vi "Puff Dose Low.vi"(0 "Save Puff Analysis file":bool, 1 "Row Number":i32, 2 "Valve Index":i32, 3 "File Extension":string=".xls", 5 "Puff Stats only?":bool, 9 "Save individual puff files":bool, 11 "Analysis info Cluster in":T2={"Colour"=0, "Inst type"=enum."Propeller anemometer", "Inst name"="", "Symbol"="", "Code name"="", "Extra Info"="", "Inst Array"=enum."PWA", "U"=0.0, "u^2"=0.0, "u^3"=0.0, "u^4"=0.0, "Skew_u"=0.0, "Kurt_u"=0.0, "Sd Error in Mean"=0.0, "% u'/U"=0.0, "X"=0.0, "Y"=0.0, "Z"=0.0, "Timescale integral Estimate"=0.0, "Sd Error in Variance"=0.0, "Calib File"=path "", "Calib Constants"=[], "Output Position"=FALSE, "Stats"=enum."None", "Av Sampling Rate"=0.0, "Av No of Samples"=0.0, "Total Meas Time (s)"=0.0, "OrigChName"="", "Max value"=0.0, "Min value"=0.0, "Req Sample Rate Hz"=0.0, "Sync Delay Time (s)"=0.0, "Ch No"=0, "Device"="", "Use Latest Calib"=FALSE, "Port"="", "Metadata Ch Names"=[], "Metadata Ch Values"=[], "Label"="", "chState"=enum."Solo", "Point Drift"=0.0, "inputConfig"=""} {"Kurt_u" format="%_3g"; "u^4" format="%_3g"; "u^3" format="%_3g"; "Sd Error in Variance" format="%_3g"; "u^2" format="%_3g"; "Sd Error in Mean" format="%_3g"; "U" format="%_3g"; "Sync Delay Time (s)" format="%.4f"; "Total Meas Time (s)" format="%_5g"; "Skew_u" format="%_3g"; "% u'/U" format="%_3g"}, 12 "Saved trace length":i32=200, 13 "FFID Index":i32, 14 "Save Av puff files":bool) -> (4 "File to Update":T1[](array[typedef]), 15 "Analysis info Cluster out":T2={"Colour"=0, "Inst type"=enum."Propeller anemometer", "Inst name"="", "Symbol"="", "Code name"="", "Extra Info"="", "Inst Array"=enum."PWA", "U"=0.0, "u^2"=0.0, "u^3"=0.0, "u^4"=0.0, "Skew_u"=0.0, "Kurt_u"=0.0, "Sd Error in Mean"=0.0, "% u'/U"=0.0, "X"=0.0, "Y"=0.0, "Z"=0.0, "Timescale integral Estimate"=0.0, "Sd Error in Variance"=0.0, "Calib File"=path "", "Calib Constants"=[], "Output Position"=FALSE, "Stats"=enum."None", "Av Sampling Rate"=0.0, "Av No of Samples"=0.0, "Total Meas Time (s)"=0.0, "OrigChName"="", "Max value"=0.0, "Min value"=0.0, "Req Sample Rate Hz"=0.0, "Sync Delay Time (s)"=0.0, "Ch No"=0, "Device"="", "Use Latest Calib"=FALSE, "Port"="", "Metadata Ch Names"=[], "Metadata Ch Values"=[], "Label"="", "chState"=enum."Solo", "Point Drift"=0.0, "inputConfig"=""} {"Kurt_u" format="%_3g"; "u^4" format="%_3g"; "u^3" format="%_3g"; "Sd Error in Variance" format="%_3g"; "u^2" format="%_3g"; "Sd Error in Mean" format="%_3g"; "U" format="%_3g"; "Sync Delay Time (s)" format="%.4f"; "Total Meas Time (s)" format="%_5g"; "Skew_u" format="%_3g"; "% u'/U" format="%_3g"})   [LabVIEW 2022 SP3]
uses:
  Controls/Analysis_info_cluster.ctl
  Controls/Inst_type.ctl
  Controls/Instrument_Array.ctl
  Controls/channelState.ctl
  File/File Update Cluster.ctl
  <vilib>/Analysis/baseanly.llb/Mean (DBL).vi
  Globals/Meas_global.vi
  Globals/Plug_in_data_global.vi
  Globals/Dynamic_call_global.ph.vi
  <vilib>/Analysis/NI_AALBase.lvlib
  <vilib>/Analysis/NI_AALPro.lvlib
panel:
  in  "Time constants cut off":dbl=3.0
  out "Numeric":dbl
  out "End Index":i32
  out "Start Index":i32
  out "Av Dose below Threshold":dbl format="%0.2f"
  out "Max Flight Time (s)":dbl
  out "Table Control":string[][](table)
  out "Minimum Dose":dbl
  out "Initial Minimum Dose":dbl
  out "Active Length":i32
  out "T1 index":i32
  out "Initial Time of Flight":dbl
  out "Output:Data File:Location":string
  out "Dose per Puff":cluster{dbl[], "Best Polynomial Fit":dbl[]}[](graph)
  out "Polynomial Coefficients":dbl[](array[numeric])
  out "Bkgnd Per Puff":cluster{dbl[], "Best Polynomial Fit":dbl[]}[](graph)
  out "Background time used (s)":dbl
  out "Delta T":dbl
  out "Bkgnd value (ppm)":dbl format="%0.2f"
  out "Puff Number":i32=51
  out "XY Graph":cluster{"Time (s)":dbl[], "Eng Values":dbl[]}[](graph)
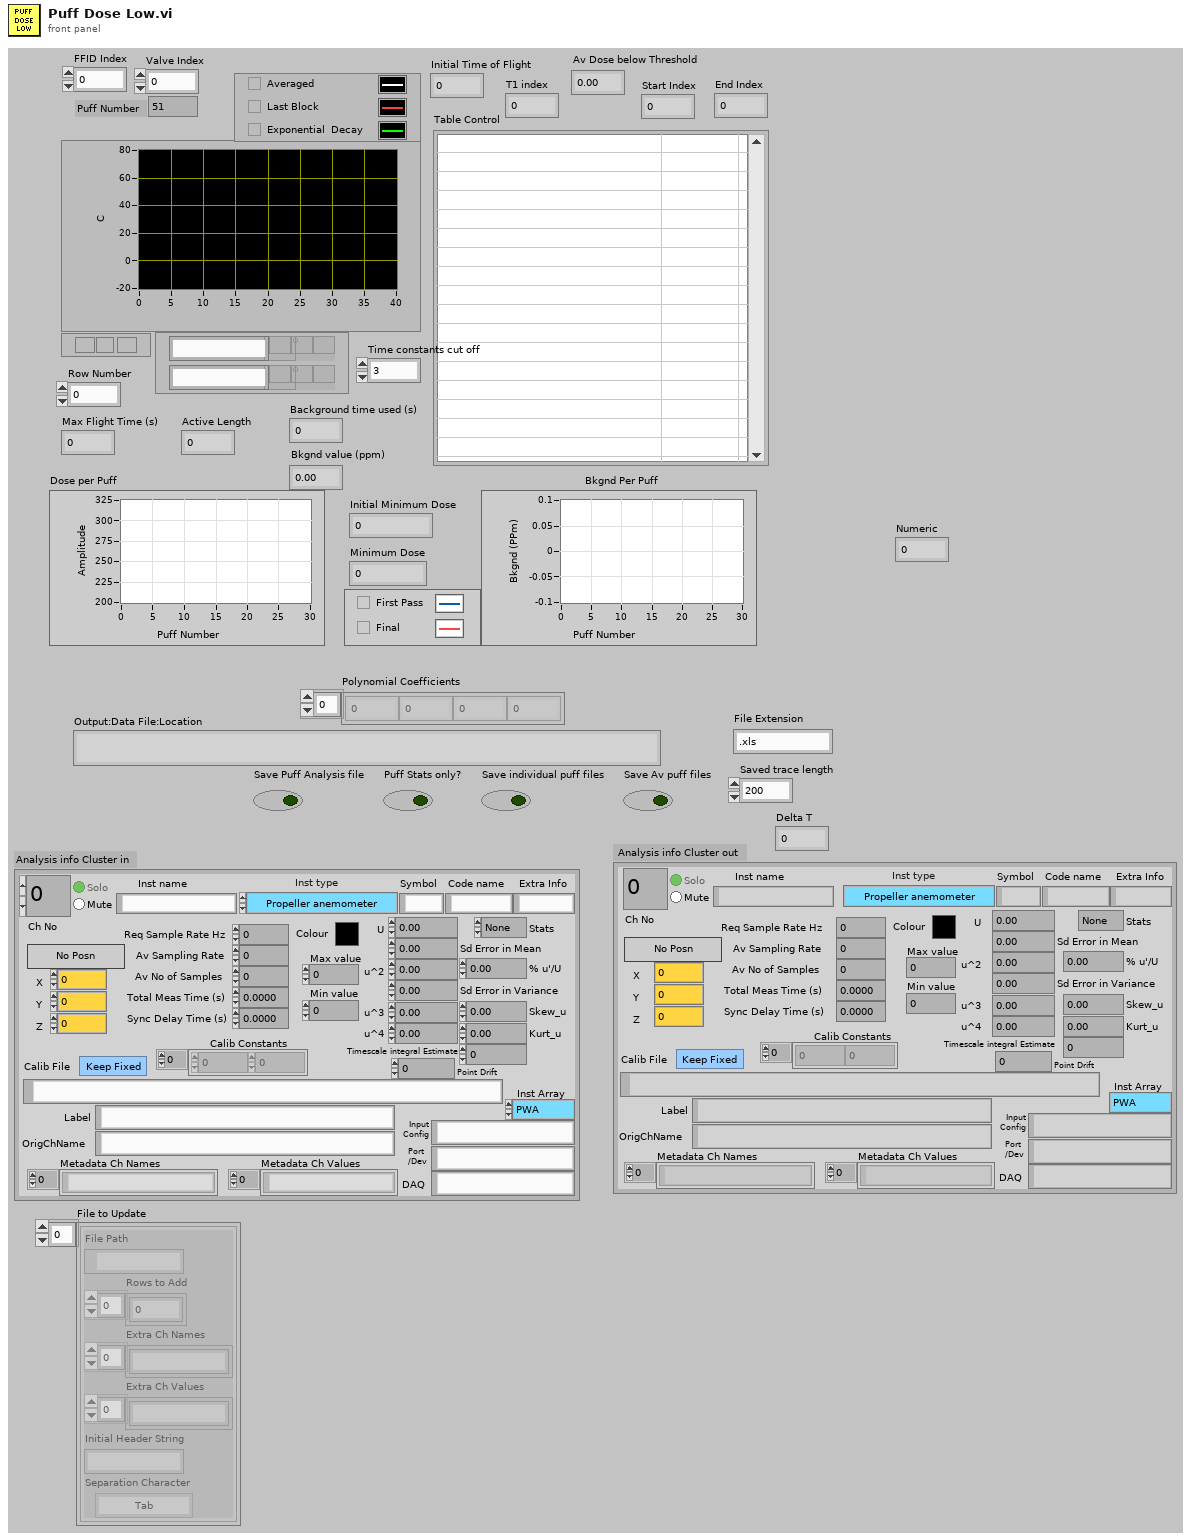
[diagram p1: front panel]
types:
  T1 = typedef "File Update Cluster.ctl" = cluster{"File Path":path, "Rows to Add":i32[], "Extra Ch Names":string[], "Extra Ch Values":string[], "Initial Header String":string, "Separation Character":enum16{"Tab", "Comma"}}
  T2 = typedef "Analysis_info_cluster.ctl" = cluster{"Colour":u32, "Inst type":T3, "Inst name":string, "Symbol":string, "Code name":string, "Extra Info":string, "Inst Array":T4, "U":dbl, "u^2":dbl, "u^3":dbl, "u^4":dbl, "Skew_u":dbl, "Kurt_u":dbl, "Sd Error in Mean":dbl, "% u'/U":dbl, "X":dbl, "Y":dbl, "Z":dbl, "Timescale integral Estimate":dbl, "Sd Error in Variance":dbl, "Calib File":path, "Calib Constants":dbl[], "Output Position":bool, "Stats":enum16{"None", "Basic", "Full"}, "Av Sampling Rate":dbl, "Av No of Samples":dbl, "Total Meas Time (s)":dbl, "OrigChName":string, "Max value":dbl, "Min value":dbl, "Req Sample Rate Hz":dbl, "Sync Delay Time (s)":dbl, "Ch No":i16, "Device":string, "Use Latest Calib":bool, "Port":string, "Metadata Ch Names":string[], "Metadata Ch Values":string[], "Label":string, "chState":T5, "Point Drift":dbl, "inputConfig":string}
  T3 = typedef "Inst_type.ctl" = enum16{"Raw voltage", "Raw with zero offsetting", "Propeller anemometer", "Pressure Transducer", "Pitot-static tube", "Hot wire", "Cross wire 1", "Cross wire 2", "Generic Linear", "Generic Polynomial", "Generic BackPoly", "Fast FID", "Thermocouple", "Cold wire", "Pulsed Wire", "LDA Vel", "LDA Tran time", "LDA Arr time", "Microphone"}
  T4 = typedef "Instrument_Array.ctl" = enum16{"PWA", "LDA", "Analogue"}
  T5 = typedef "channelState.ctl" = enum32{"No Selection", "Solo", "Mute"}
  T6 = enum16{"Save no data", "Save data in new files", "Save data in existing files"}
  T7 = typedef "Time_Trace_Cluster.ctl" = cluster{"Weighting":dbl[], "Voltage":dbl[], "Eng Values":dbl[]}
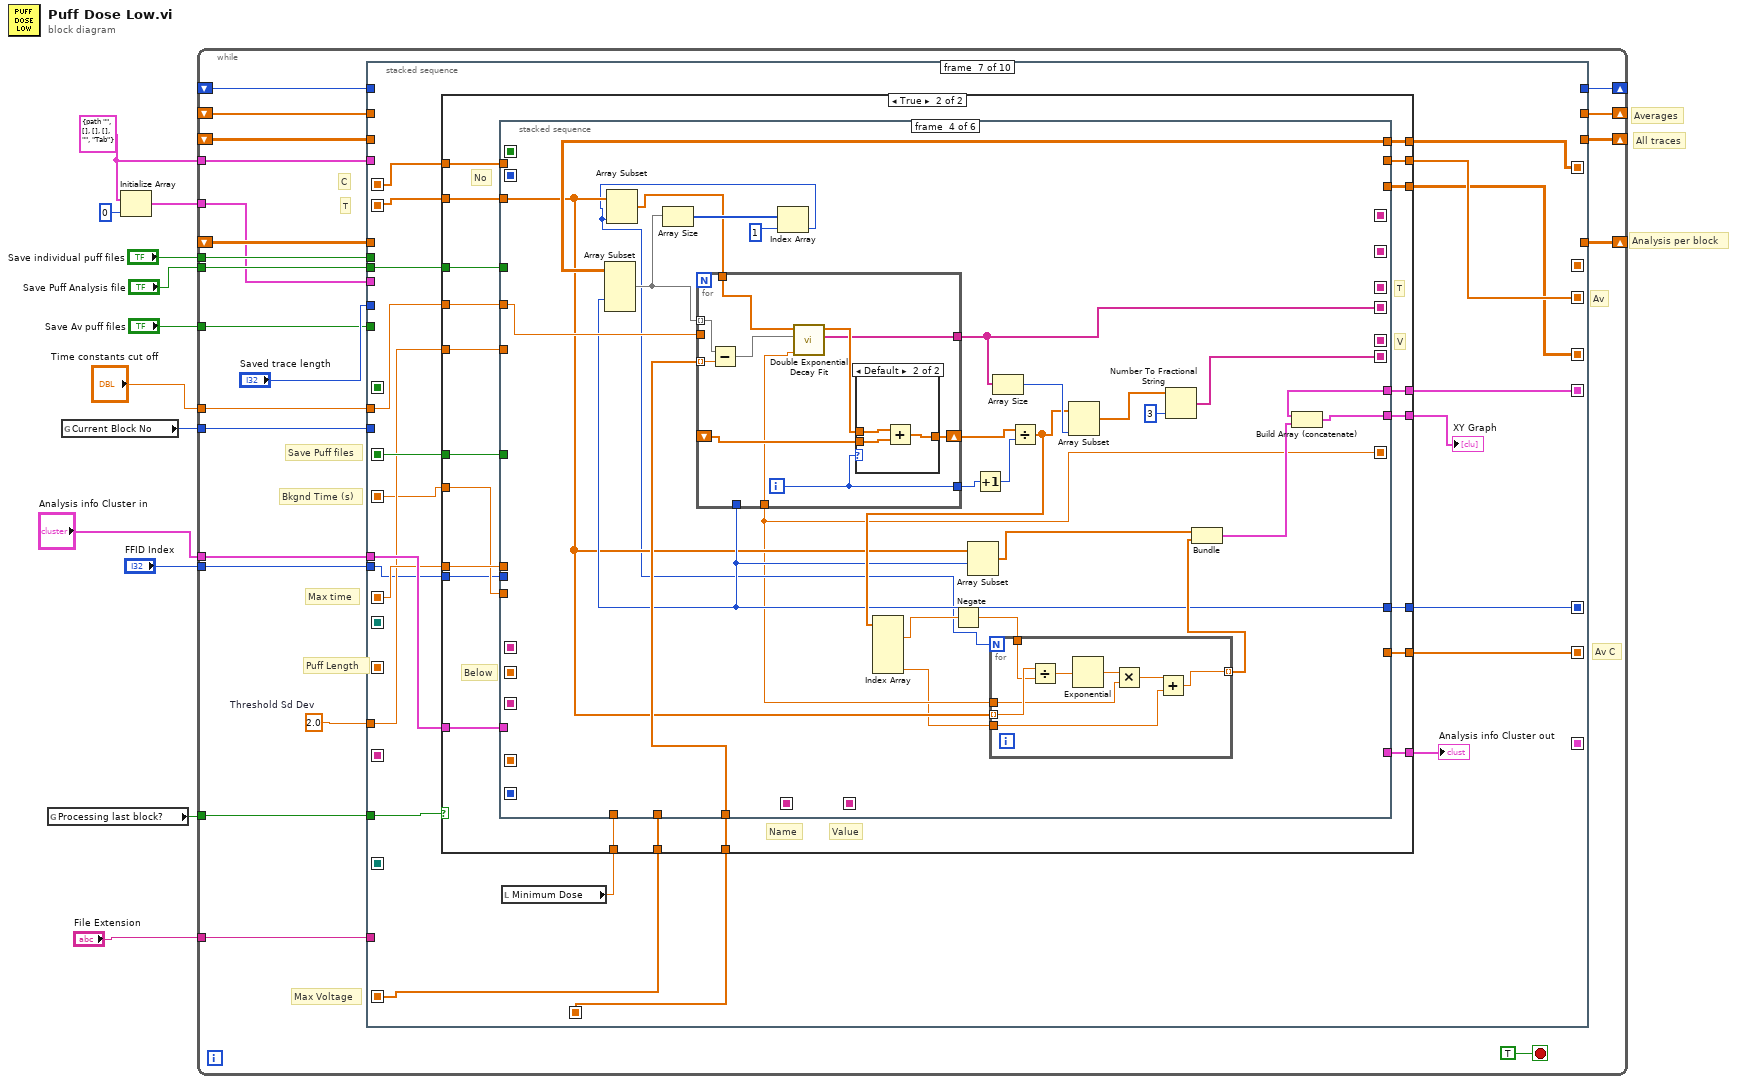
[diagram p0: block diagram]
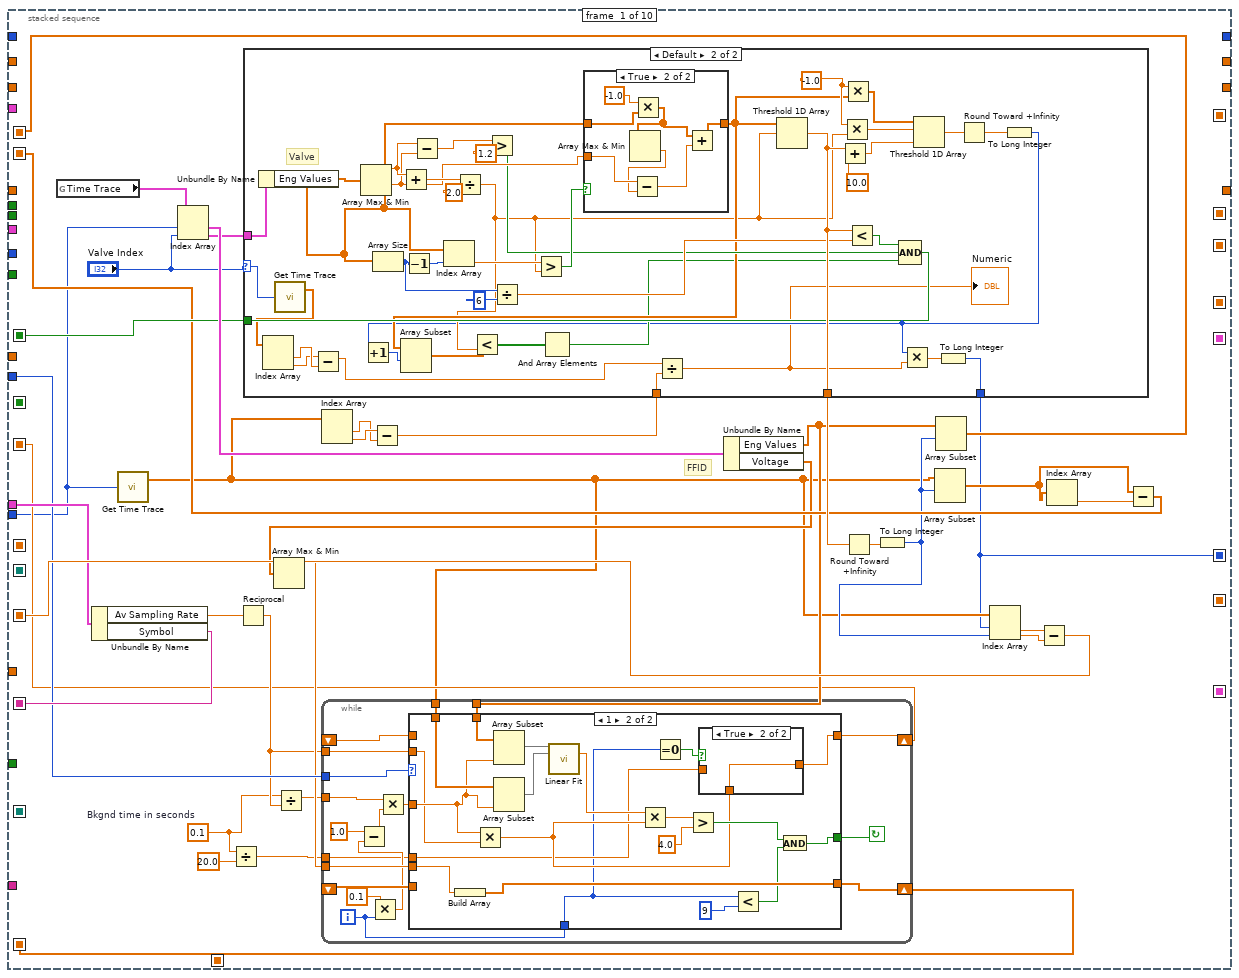
[diagram p2: hidden frame]
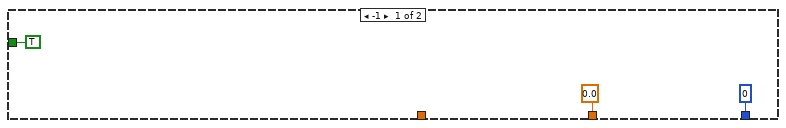
[diagram p3: hidden frame]
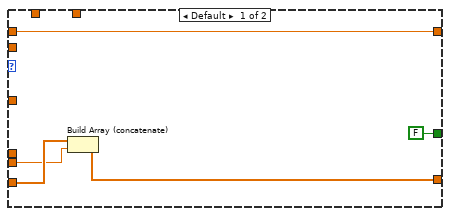
[diagram p5: hidden frame]
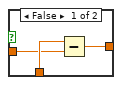
[diagram p6: hidden frame]
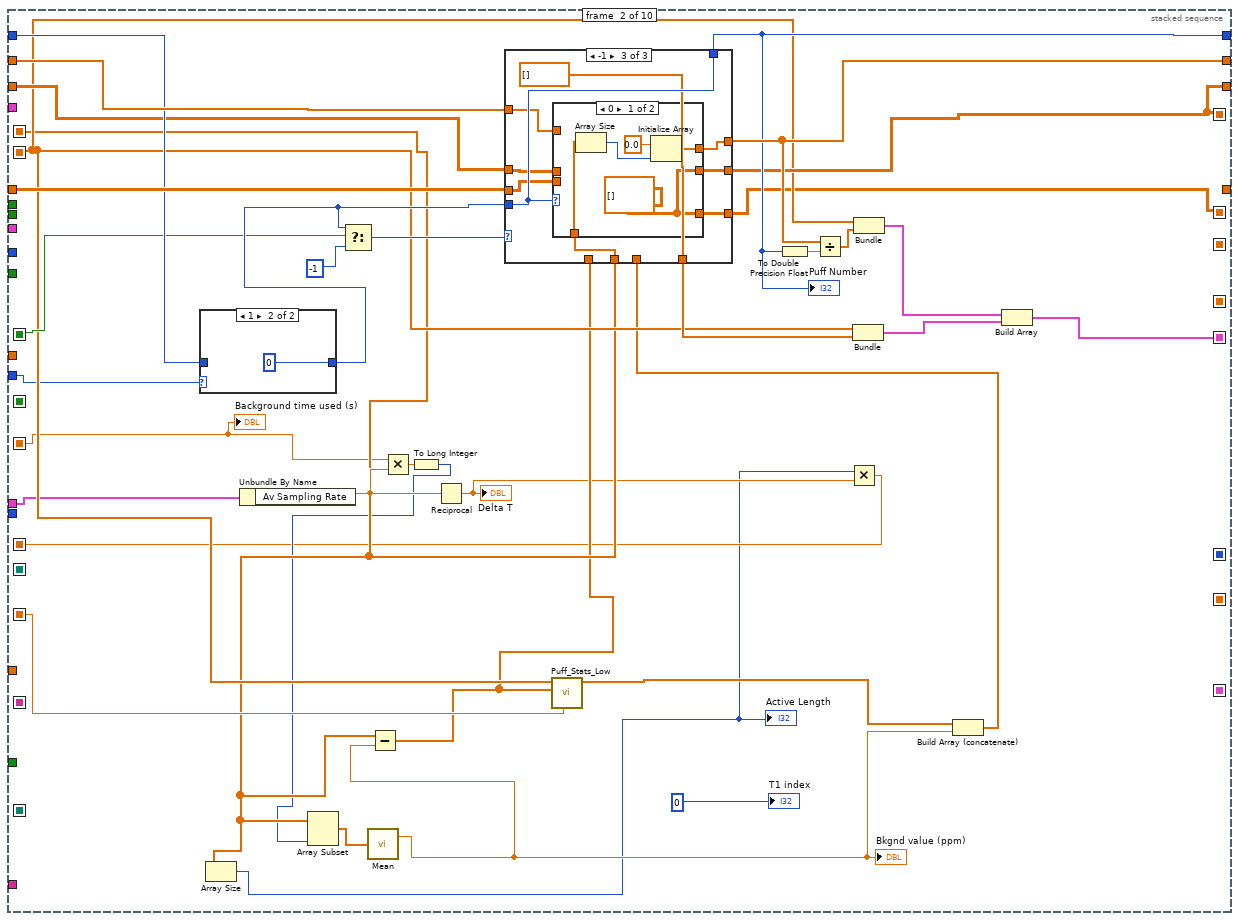
[diagram p7: hidden frame]
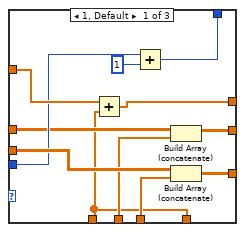
[diagram p9: hidden frame]
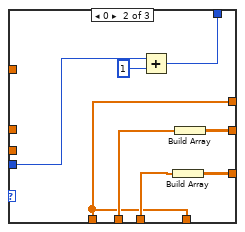
[diagram p10: hidden frame]
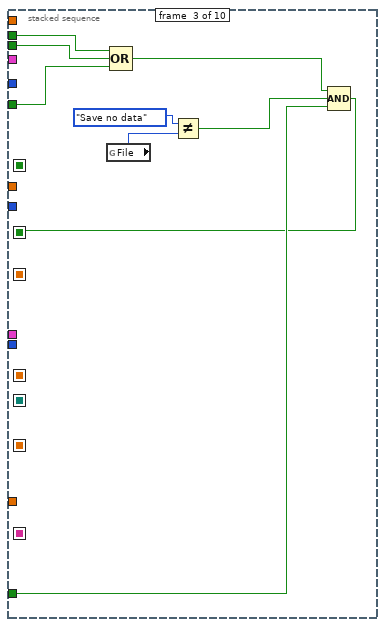
[diagram p12: hidden frame]
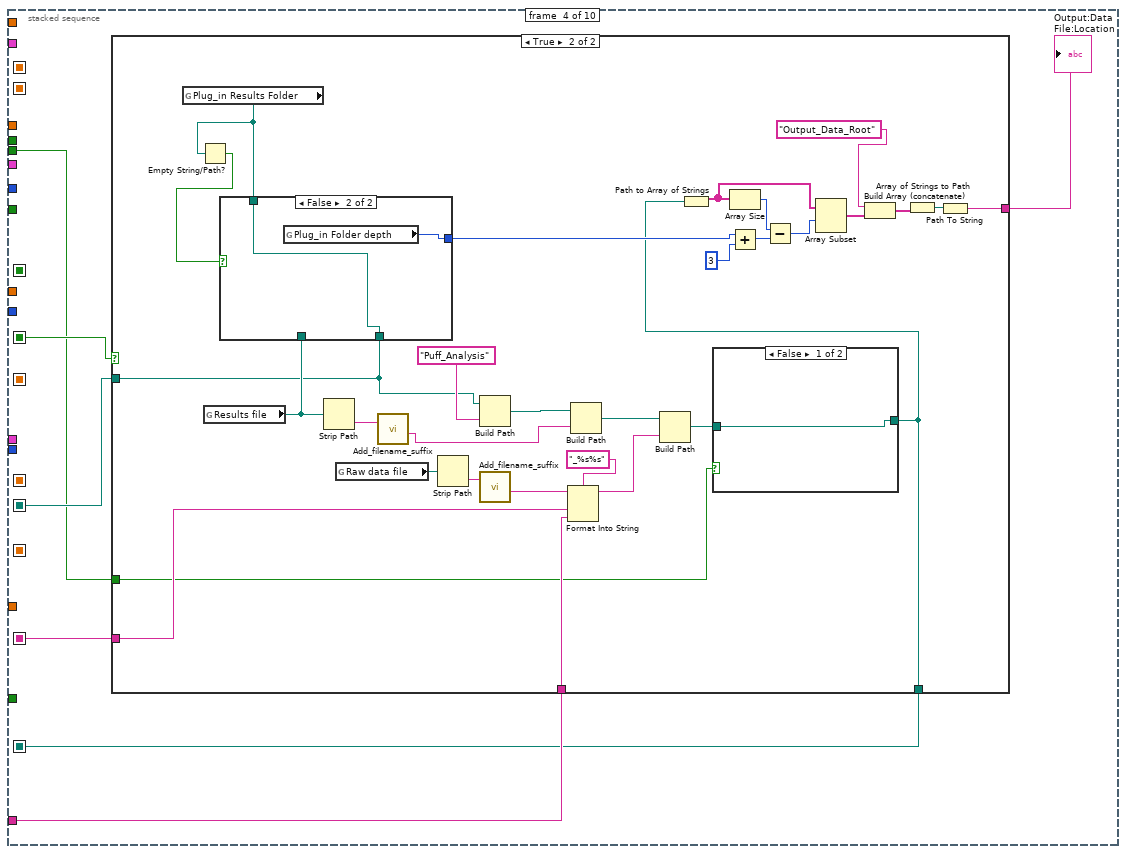
[diagram p13: hidden frame]
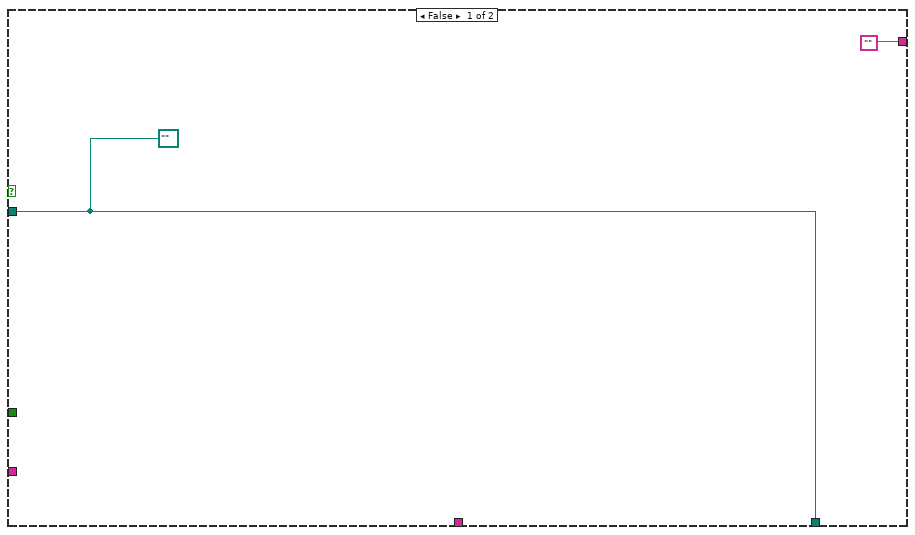
[diagram p14: hidden frame]
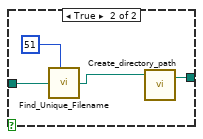
[diagram p15: hidden frame]
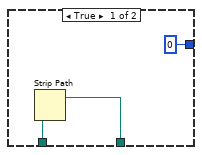
[diagram p16: hidden frame]
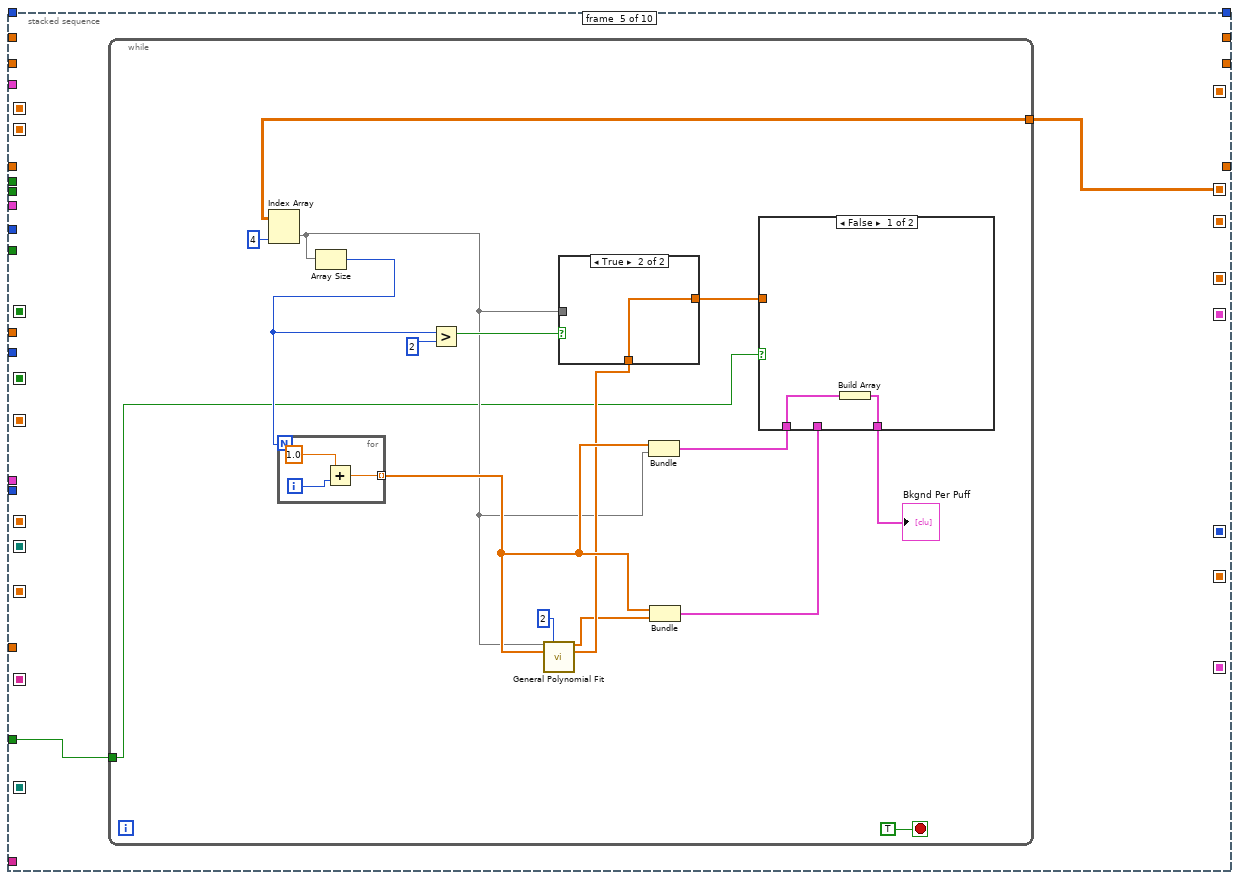
[diagram p17: hidden frame]
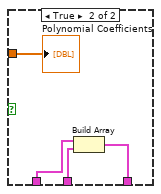
[diagram p18: hidden frame]
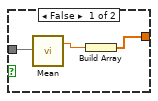
[diagram p19: hidden frame]
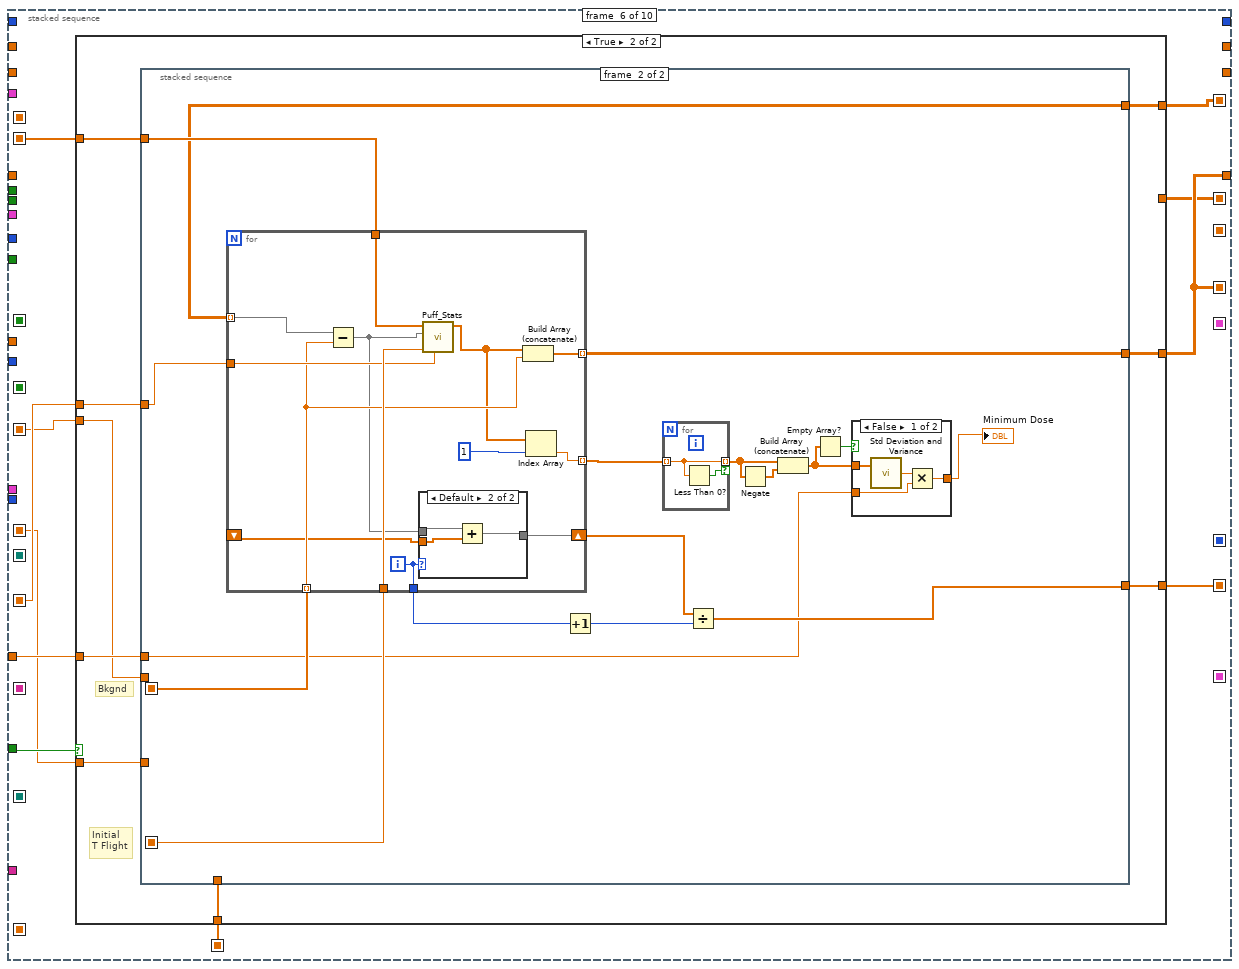
[diagram p20: hidden frame]
diagram:
  w2 = T1 {"File Path"=path "", "Rows to Add"=[], "Extra Ch Names"=[], "Extra Ch Values"=[], "Initial Header String"="", "Separation Character"=enum."Tab"} ("File to Update")
  # "Averages"
  # "All traces"
  # "Analysis per block"
  n1 = global read "Meas_global.vi" "Processing last block?"() -> (w11:bool)
  n2 = global read "Meas_global.vi" "Current Block No"() -> (w7:i32)
  n3 = Initialize Array(w2, 0 ("dimension size")) -> (w3:T1[])
  n4 = while {
    shift-right: [w32] -> _
    shift-left: _ -> [w34]
    shift-right: [w30] -> _
    shift-left: _ -> [w31]
    shift-right: [w28] -> _
    shift-left: _ -> [w29]
    shift-right: [w27] -> _
    shift-left: _ -> [w26]
    tunnel: "Save Puff Analysis file" -> [w25]
    tunnel: w11 -> [w24]
    tunnel: "FFID Index" -> [w23]
    tunnel: "Analysis info Cluster in" -> [w22]
    tunnel: "File Extension" -> [w21]
    tunnel: w7 -> [w19]
    tunnel: "Save Av puff files" -> [w17]
    tunnel: "Save individual puff files" -> [w16]
    tunnel: w3 -> [w15]
    tunnel: w2 -> [w14]
    tunnel: "Time constants cut off" -> [w13]
    stop <- TRUE stop-if-true
    w18 = 2.0  # Threshold Sd Dev
    # "Bkgnd Time (s)"
    # "Max time"
    # "Av C"
    # "Max Voltage"
    # "Av"
    # "Save Puff files"
    # "Puff Length"
    # "T"
    # "C"
    n5 = stacked-sequence {
      seq-local: [_ w178 _ _ _ _ _ _ _ _] -> [_ _ _ _ w303 w338 _ w698 _ _]
      seq-local: [w60 _ _ _ _ _ _ _ _ _] -> [_ w177 _ _ _ _ w451 _ _ _]
      seq-local: [w61 _ _ _ _ _ _ _ _ _] -> [_ w186 _ _ _ w341 w464 _ w728 _]
      seq-local: [w58 _ _ _ _ _ _ _ _ _] -> [_ w185 _ _ _ w340 _ _ _ _]
      seq-local: [w64 _ _ _ _ _ _ _ _ _] -> [_ w192 _ _ _ _ _ _ _ _]
      seq-local: [_ w188 _ _ _ _ _ _ _ _] -> [_ _ _ _ _ w342 w447 _ w729 _]
      seq-local: [_ _ w248 _ _ _ _ _ _ _] -> [_ _ _ w254 _ _ w460 _ w727 _]
      seq-local: [w59 _ _ _ _ _ _ _ _ _] -> [_ _ _ w258 _ _ _ _ w726 _]
      seq-local: [_ _ _ _ _ _ w463 _ _ _] -> [_ _ _ _ _ _ _ _ w724 _]
      seq-local: [_ _ _ w257 _ _ _ _ _ _] -> [_ _ _ _ _ _ _ _ w721 _]
      seq-local: [_ _ _ w255 _ _ _ _ _ _] -> [_ _ _ _ _ _ _ _ w722 _]
      seq-local: [_ _ _ _ _ _ _ _ w720 _] -> [_ _ _ _ _ _ _ _ _ w1015]
      seq-local: [w51 _ _ _ _ _ _ _ _ _] -> [_ _ _ _ _ _ w459 _ _ _]
      seq-local: [_ _ _ _ _ w339 _ _ _ _] -> [_ _ _ _ _ _ w458 w708 w718 _]
      seq-local: [_ _ _ _ _ w337 _ _ _ _] -> [_ _ _ _ _ _ w445 _ _ _]
      seq-local: [_ _ _ _ _ w336 _ _ _ _] -> [_ _ _ _ _ _ w456 _ w717 _]
      seq-local: [_ w172 _ _ _ _ _ _ _ _] -> [_ _ _ _ _ w334 w455 _ _ _]
      seq-local: [w45 _ _ _ _ _ _ _ _ _] -> [_ w170 _ _ _ w333 w453 _ _ _]
      seq-local: [w35 _ _ _ _ _ _ _ _ _] -> [_ _ _ _ _ _ w450 _ _ _]
      seq-local: [_ w169 _ _ _ _ _ _ _ _] -> [_ _ _ _ _ _ w449 _ _ _]
      tunnel: w34 -> [_ w198 _ _ _ _ _ _ _ _]
      tunnel: [_ w203 _ _ _ _ _ _ _ _] -> w32
      tunnel: w31 -> [_ w199 _ _ _ _ _ _ _ _]
      tunnel: [_ _ _ _ _ w339 _ _ _ _] -> w30
      tunnel: w29 -> [_ w197 _ _ _ _ _ _ _ _]
      tunnel: [_ w196 _ _ _ _ _ _ _ _] -> w28
      tunnel: [_ w188 _ _ _ _ _ _ _ _] -> w27
      tunnel: w26 -> [_ w190 _ _ _ _ _ _ _ _]
      tunnel: w25 -> [_ _ w246 w253 _ _ w466 _ w714 _]
      tunnel: w24 -> [_ _ w249 _ w302 w343 w465 _ _ _]
      tunnel: w17 -> [_ _ w245 _ _ _ _ _ w725 _]
      tunnel: w23 -> [w41 _ _ _ _ _ w452 _ _ _]
      tunnel: w22 -> [w54 w180 _ _ _ _ w462 _ w713 _]
      tunnel: w21 -> [_ _ _ w259 _ _ _ _ w723 _]
      tunnel: "Saved trace length" -> [_ _ _ _ _ _ _ _ w719 _]
      tunnel: w19 -> [w53 w179 _ _ _ _ _ _ _ _]
      tunnel: w18 -> [_ _ _ _ _ w335 w454 _ _ _]
      tunnel: w16 -> [_ _ w247 _ _ _ _ _ w716 _]
      tunnel: w15 -> [_ _ _ _ _ _ _ _ w715 _]
      tunnel: w14 -> [_ _ _ _ _ _ _ _ w712 _]
      tunnel: w13 -> [_ _ _ _ _ _ w446 _ _ _]
      frame #0 {
        w44 = 0.1  # Bkgnd time in seconds
        # "FFID"
        n6 = global read "Meas_global.vi" "Time Trace"() -> (w69:T7[])
        n7 = Unbundle By Name(w54) -> ("Av Sampling Rate"=w48:dbl, "Symbol"=w59:string)
        n8 = call "Get Time Trace.vi"("Channel Index"=w41) -> ("Time (s)"=w39:dbl[])  [unwired: 1 out]
        n9 = Index Array(array=w69, index #1=w41, index #2="Valve Index") -> (element #1=w68:T7, element #2=w67:T7)
        n10 = Divide(x=w44, y=20.0) -> (x/y=w42:dbl)
        n11 = Reciprocal(x=w48) -> (1/x=w46:dbl)
        n12 = Divide(x=w44, y=w46) -> (x/y=w47:dbl)
        n13 = Index Array(array=w39) -> (element #1=w37:dbl, element #2=w38:dbl)  [unwired: 2 in]
        n14 = Subtract(x=w38, y=w37) -> (x-y=w36:dbl)
        n15 = case shown="Default" "Valve Index" {
          selector: "Valve Index" -> [_ w82]
          tunnel: w67 -> [_ w113]
          tunnel: [0.0 w98] -> w65
          tunnel: [TRUE w92] -> w64
          tunnel: [0 w74] -> w35
          tunnel: w36 -> [_ w77]
          frame -1 {
          }
          frame Default {
            w108 = -1.0
            # "Valve"
            n16 = Unbundle By Name(w113) -> ("Eng Values"=w91:dbl[])
            n17 = call "Get Time Trace.vi"("Channel Index"=w82) -> ("Time (s)"=w79:dbl[])  [unwired: 1 out]
            n18 = Index Array(array=w79) -> (element #1=w81:dbl, element #2=w80:dbl)  [unwired: 2 in]
            n19 = Subtract(x=w80, y=w81) -> (x-y=w78:dbl)
            n20 = Array Max & Min(array=w91) -> (max value=w102:dbl, min value=w101:dbl)  [unwired: 2 out]
            n21 = Array Size(array=w91) -> (size(s)=w97:i32)
            n22 = Add(x=w102, y=w101) -> (x+y=w112:dbl)
            n23 = Decrement(x=w97) -> (x-1=w106:i32)
            n24 = Subtract(x=w102, y=w101) -> (x-y=w100:dbl)
            n25 = Index Array(array=w91, index=w106) -> (element=w105:dbl)
            n26 = Divide(x=w112, y=2.0) -> (x/y=w87:dbl)
            n27 = Greater?(x=w100, y=1.2) -> (0:w93:bool)
            n28 = Divide(x=w97, y=6) -> (x/y=w95:dbl)
            n29 = Greater?(x=w105, y=w87) -> (0:w104:bool)
            n30 = case shown="True" w104 {
              tunnel: w91 -> [w114 w120]
              tunnel: [w114 w115] -> w89
              tunnel: w101 -> [_ w119]
              frame False {
              }
              frame True {
                n31 = Multiply(x=-1.0, y=w120) -> (x*y=w116:dbl[])
                n32 = Array Max & Min(array=w116) -> (min value=w118:dbl)  [unwired: 3 out]
                n33 = Subtract(x=w119, y=w118) -> (x-y=w117:dbl)
                n34 = Add(x=w116, y=w117) -> (x+y=w115:dbl[])
              }
            }
            n35 = Divide(x=w78, y=w77) -> (x/y=w73:dbl)
            "Numeric" <- w73
            n36 = Threshold 1D Array(2:w87, 3:w89) -> (0:w98:dbl)  [unwired: 1 in]
            n37 = Add(x=w98, y=10.0) -> (x+y=w110:dbl)
            n38 = Multiply(x=w108, y=w87) -> (x*y=w107:dbl)
            n39 = Multiply(x=w108, y=w89) -> (x*y=w103:dbl[])
            n40 = Less?(x=w98, y=w95) -> (x < y?=w94:bool)
            n41 = Threshold 1D Array(1:w110, 2:w107, 3:w103) -> (0:w84:dbl)
            n42 = Round Toward +Infinity(x=w84) -> (ceil(x): smallest int >= x=w83:dbl)
            n43 = To Long Integer(number=w83) -> (32bit integer=w76:i32)
            n44 = Increment(x=w76) -> (x+1=w90:i32)
            n45 = Array Subset(array=w89, index=w90) -> (w88:dbl[])  [unwired: 1 in]
            n46 = Less?(x=w88, y=w87) -> (x < y?=w86:bool[])
            n47 = And Array Elements(Boolean array=w86) -> (logical AND=w85:bool)
            n48 = Compound Arithmetic op=AND(w94, w93, w85) -> (w92:bool)
            n49 = Multiply(x=w76, y=w73) -> (x*y=w75:dbl)
            n50 = To Long Integer(number=w75) -> (32bit integer=w74:i32)
          }
        }
        n51 = Unbundle By Name(w68) -> ("Eng Values"=w49:dbl[], "Voltage"=w50:dbl[])
        n52 = Array Max & Min(array=w50) -> (max value=w52:dbl)  [unwired: 3 out]
        n53 = while {
          shift-right: [w137] -> w51
          shift-left: _ -> [w136]
          tunnel: w53 -> [w139]
          tunnel: w52 -> [w138]
          shift-right: [w135] -> w45
          shift-left: _ -> [w134]
          tunnel: w49 -> [w133]
          tunnel: w47 -> [w128]
          tunnel: w39 -> [w126]
          tunnel: w46 -> [w125]
          tunnel: w42 -> [w122]
          i -> [w123]
          stop <- w124 continue-if-true
          n54 = Multiply(x=0.1, y=w123) -> (x*y=w130:dbl)
          n55 = Subtract(x=1.0, y=w130) -> (x-y=w129:dbl)
          n56 = Multiply(x=w128, y=w129) -> (x*y=w127:dbl)
          n57 = case shown="1" w139 {
            tunnel: w138 -> [w143 w164]
            tunnel: [w142 w163] -> w137
            tunnel: w136 -> [w144 _]
            tunnel: [w141 w148] -> w135
            tunnel: w134 -> [w141 _]
            tunnel: w133 -> [_ w162]
            tunnel: w127 -> [_ w158]
            tunnel: w126 -> [_ w160]
            tunnel: w125 -> [_ w157]
            tunnel: [FALSE w151] -> w124
            tunnel: w123 -> [_ w146]
            tunnel: w122 -> [_ w147]
            frame Default {
              n58 = Build Array (concatenate)(w144, w143) -> (w142:dbl[])
            }
            frame 1 {
              n59 = Build Array(w164) -> (w163:dbl[])
              n60 = Multiply(x=w158, y=w157) -> (x*y=w149:dbl)
              n61 = Array Subset(array=w162, length=w158) -> (w161:dbl[])  [unwired: 1 in]
              n62 = Array Subset(array=w160, length=w158) -> (w159:dbl[])  [unwired: 1 in]
              n63 = call <vilib>:"Linear Fit.vi"("Y"=w161, "X"=w159) -> ("slope"=w156:dbl)  [unwired: 9 in, 4 out]
              n64 = Multiply(x=w156, y=w149) -> (x*y=w155:dbl)
              n65 = Equal To 0?(x=w146) -> (x = 0?=w145:bool)
              n66 = Greater?(x=w155, y=4.0) -> (0:w152:bool)
              n67 = case shown="True" w145 {
                tunnel: w149 -> [w167 w168]
                tunnel: [w166 w168] -> w148
                tunnel: w147 -> [w165 _]
                frame False {
                  n68 = Subtract(x=w167, y=w165) -> (x-y=w166:dbl)
                }
                frame True {
                }
              }
              n69 = Less?(x=w146, y=9) -> (x < y?=w150:bool)
              n70 = And(x=w152, y=w150) -> (x .and. y?=w151:bool)
            }
          }
        }
        n71 = Round Toward +Infinity(x=w65) -> (ceil(x): smallest int >= x=w66:dbl)
        n72 = To Long Integer(number=w66) -> (32bit integer=w55:i32)
        n73 = Array Subset(array=w39, index=w55) -> (w62:dbl[])  [unwired: 1 in]
        n74 = Array Subset(array=w49, index=w55) -> (w60:dbl[])  [unwired: 1 in]
        n75 = Index Array(array=w39, index #1=w35, index #2=w55) -> (element #1=w57:dbl, element #2=w56:dbl)
        n76 = Subtract(x=w57, y=w56) -> (x-y=w58:dbl)
        n77 = Index Array(array=w62) -> (element=w63:dbl)  [unwired: 1 in]
        n78 = Subtract(x=w62, y=w63) -> (x-y=w61:dbl[])
      }
      frame #1 {
        n79 = case shown="1" w179 {
          tunnel: [w205 0] -> w195
          tunnel: w197 -> [w205 _]
          frame 2, Default {
          }
          frame 1 {
          }
        }
        n80 = Array Size(array=w177) -> (size(s)=w171:i32)
        "Active Length" <- w171
        n81 = Unbundle By Name(w180) -> ("Av Sampling Rate"=w200:dbl)
        n82 = Select(t=w195, s=w192, f=-1) -> (s? t:f=w193:i32)
        n83 = Multiply(x=w170, y=w200) -> (x*y=w187:dbl)
        n84 = To Long Integer(number=w187) -> (32bit integer=w173:i32)
        n85 = Array Subset(array=w177, length=w173) -> (w175:dbl[])  [unwired: 1 in]
        n86 = call-poly <vilib>:"Mean.vi"("X"=w175) -> ("mean"=w183:dbl)  [unwired: 1 out]
        "Bkgnd value (ppm)" <- w183
        n87 = Subtract(x=w177, y=w183) -> (x-y=w176:dbl[])
        n88 = Reciprocal(x=w200) -> (1/x=w174:dbl)
        "Delta T" <- w174
        n89 = call "Puff_Stats_Low.vi"("Puff release time (s)"=w185, "Concentrations"=w176, "Time (s)"=w186) -> ("Stats"=w184:dbl[])  [unwired: 8 in]
        n90 = Multiply(x=w171, y=w174) -> (x*y=w172:dbl)
        n91 = Build Array (concatenate)(w184, w183) -> (w182:dbl[])
        n92 = case shown="-1" w193 {
          tunnel: [w217 w219 w234] -> w203
          tunnel: w198 -> [w218 _ w233]
          tunnel: w182 -> [w216 w226 _]
          tunnel: [w215 w225 w229] -> w178
          tunnel: w199 -> [w214 _ w232]
          tunnel: w195 -> [w211 w224 w235]
          tunnel: [w212 w222 w235] -> w196
          tunnel: w177 -> [w209 w221 w231]
          tunnel: [w207 w219 dbl[] []] -> w191
          tunnel: [w208 w220 w228] -> w188
          tunnel: w190 -> [w210 _ w227]
          tunnel: w176 -> [w207 w219 _]
          frame 1, Default {
            n93 = Add(x=w218, y=w207) -> (x+y=w217:dbl[])
            n94 = Add(x=w211, y=1) -> (x+y=w212:i32)
            n95 = Build Array (concatenate)(w210, w209) -> (w208:dbl[][])
            n96 = Build Array (concatenate)(w214, w216) -> (w215:dbl[][])
          }
          frame 0 {
            n97 = Add(x=w224, y=1) -> (x+y=w222:i32)
            n98 = Build Array(w226) -> (w225:dbl[][])
            n99 = Build Array(w221) -> (w220:dbl[][])
          }
          frame -1 {
            n100 = case shown="0" w235 {
              tunnel: w231 -> [w240 _]
              tunnel: [w237 w243] -> w234
              tunnel: [w236 w242] -> w229
              tunnel: w233 -> [_ w243]
              tunnel: w232 -> [_ w242]
              tunnel: [w236 w241] -> w228
              tunnel: w227 -> [_ w241]
              frame 0 {
                w236 = dbl[][] []
                n101 = Array Size(array=w240) -> (size(s)=w239:i32)
                n102 = Initialize Array(0.0 ("element"), w239) -> (w237:dbl[])
              }
              frame 1, Default {
              }
            }
          }
        }
        "Puff Number" <- w196
        n103 = To Double Precision Float(number=w196) -> (double precision float=w204:dbl)
        n104 = Divide(x=w203, y=w204) -> (x/y=w189:dbl[])
        n105 = Bundle(w186, w191) -> (w202:cluster{dbl[], dbl[]})  [unwired: 1 in]
        n106 = Bundle(w186, w189) -> (w201:cluster{dbl[], dbl[]})  [unwired: 1 in]
        n107 = Build Array(w201, w202) -> (w169:cluster{dbl[], dbl[]}[])
        "Background time used (s)" <- w170
        "T1 index" <- 0 ("Active Length")
      }
      frame #2 {
        n108 = global read "Meas_global.vi" "File"() -> (w252:T6)
        n109 = Compound Arithmetic op=OR(w247, w246, w245) -> (w244:bool)
        n110 = Not Equal?(x=T6."Save no data" ("File"), y=w252) -> (x != y?=w250:bool)
        n111 = Compound Arithmetic op=AND(w244, w250, w249) -> (w248:bool)
      }
      frame #3 {
        n112 = case shown="True" w254 {
          tunnel: w259 -> [_ w267]
          tunnel: w258 -> [_ w266]
          tunnel: [w261 w265] -> w257
          tunnel: ["" w264] -> w256
          tunnel: [w261 w263] -> w255
          tunnel: w253 -> [_ w262]
          frame False {
            w261 = path "" ("Plug_in Results Folder")
          }
          frame True {
            n113 = global read "Plug_in_data_global.vi" "Plug_in Results Folder"() -> (w281:path)
            n114 = Empty String/Path?(string/path=w281) -> (empty?=w282:bool)
            n115 = global read "Meas_global.vi" "Results file"() -> (w280:path)
            n116 = case shown="False" w282 {
              tunnel: w281 -> [_ w301]
              tunnel: [w299 w301] -> w265
              tunnel: w280 -> [w298 _]
              tunnel: [0 ("Plug_in Folder depth") w300] -> w272
              frame True {
                n117 = Strip Path(path=w298) -> (stripped path=w299:path)  [unwired: 1 out]
              }
              frame False {
                n118 = global read "Plug_in_data_global.vi" "Plug_in Folder depth"() -> (w300:i32)
              }
            }
            n119 = Strip Path(path=w280) -> (name=w286:string)  [unwired: 1 out]
            n120 = global read "Meas_global.vi" "Raw data file"() -> (w290:path)
            n121 = call "Add_filename_suffix.vi"("Filename"=w286) -> ("Base name"=w284:string)  [unwired: 1 in, 3 out]
            n122 = Strip Path(path=w290) -> (name=w291:string)  [unwired: 1 out]
            n123 = Build Path(base path=w265, name or relative path="Puff_Analysis") -> (appended path=w285:path)
            n124 = call "Add_filename_suffix.vi"("Filename"=w291) -> ("Base name"=w287:string)  [unwired: 1 in, 3 out]
            n125 = Format Into String(format string="_%s%s", initial string=w287, w266, w267) -> (resulting string=w283:string)  [unwired: 1 in, 1 out]
            n126 = Build Path(base path=w285, name or relative path=w284) -> (appended path=w289:path)
            n127 = Build Path(base path=w289, name or relative path=w283) -> (appended path=w288:path)
            n128 = case shown="False" w262 {
              tunnel: w288 -> [w292 w296]
              tunnel: [w292 w293] -> w263
              frame False {
              }
              frame True {
                n129 = call "Find_Unique_Filename.vi"("Path In"=w296, "Max Length (31)"=51) -> ("Unique Path Out"=w295:path)  [unwired: 1 in]
                n130 = call "Create_directory_path.vi"("Path name"=w295) -> ("Path name Out"=w293:path)  [unwired: 2 in, 1 out]
              }
            }
            n131 = Path to Array of Strings(0:w263) -> (2:w278:string[])  [unwired: 1 out]
            n132 = Array Size(array=w278) -> (size(s)=w279:i32)
            n133 = Add(x=w272, y=3) -> (x+y=w273:i32)
            n134 = Subtract(x=w279, y=w273) -> (x-y=w277:i32)
            n135 = Array Subset(array=w278, index=w277) -> (w275:string[])  [unwired: 1 in]
            n136 = Build Array (concatenate)("Output_Data_Root", w275) -> (w274:string[])
            n137 = Array of Strings to Path(0:w274) -> (2:w276:path)  [unwired: 1 in]
            n138 = Path To String(path=w276) -> (string=w264:string)
          }
        }
        "Output:Data File:Location" <- w256
      }
      frame #4 {
        n139 = while {
          tunnel: w303 -> [w311]
          tunnel: w302 -> [w307]
          stop <- TRUE stop-if-true
          n140 = Index Array(array=w311, index (col)=4 ("disabled index (col)")) -> (element=w314:dbl[])  [unwired: 1 in]
          n141 = Array Size(array=w314) -> (size(s)=w317:i32)
          n142 = for {
            N: w317 -> [_]
            tunnel: [w330] -> w318 mode=indexing
            i -> [w332]
            n143 = Add(x=1.0, y=w332) -> (x+y=w330:dbl)
          }
          n144 = Greater?(x=w317, y=2) -> (0:w316:bool)
          n145 = call <vilib>:"General Polynomial Fit.vi"("Y"=w314, "polynomial order"=2, "X"=w318) -> ("Best Polynomial Fit"=w310:dbl[], "Polynomial Coefficients"=w315:dbl[])  [unwired: 9 in, 2 out]
          n146 = case shown="True" w316 {
            tunnel: [w326 w329] -> w304
            tunnel: w315 -> [_ w329]
            tunnel: w314 -> [w328 _]
            frame False {
              n147 = call-poly <vilib>:"Mean.vi"("X"=w328) -> ("mean"=w327:dbl)  [unwired: 1 out]
              n148 = Build Array(w327) -> (w326:dbl[])
            }
            frame True {
            }
          }
          n149 = Bundle(w318, w314) -> (w308:cluster{dbl[], dbl[]})  [unwired: 1 in]
          n150 = Bundle(w318, "Best Polynomial Fit"=w310) -> (w305:cluster{dbl[], "Best Polynomial Fit":dbl[]})  [unwired: 1 in]
          n151 = case shown="False" w307 {
            tunnel: w308 -> [w321 w324]
            tunnel: [w320 w323] -> w306
            tunnel: w305 -> [_ w325]
            tunnel: w304 -> [_ w322]
            frame False {
              n152 = Build Array(w321) -> (w320:cluster{dbl[], dbl[]}[])
            }
            frame True {
              n153 = Build Array(w324, w325) -> (w323:cluster{dbl[], "Best Polynomial Fit":dbl[]}[])
              "Polynomial Coefficients" <- w322
            }
          }
          "Bkgnd Per Puff" <- w306
        }
      }
      frame #5 {
        n154 = case shown="True" w343 {
          tunnel: w342 -> [_ w355]
          tunnel: w341 -> [_ w354]
          tunnel: w340 -> [_ w353]
          tunnel: [w346 w352] -> w339
          tunnel: w338 -> [w346 _]
          tunnel: [dbl[] [] w351] -> w337
          tunnel: [dbl[] [] w350] -> w336
          tunnel: w335 -> [_ w349]
          tunnel: w334 -> [_ w348]
          tunnel: w333 -> [_ w347]
          frame False {
          }
          frame True {
            # "Initial\nT Flight"
            # "Bkgnd"
            n155 = stacked-sequence {
              seq-local: [w370 _] -> [_ w419]
              seq-local: [w359 _] -> [_ w417]
              tunnel: w355 -> [w369 w415]
              tunnel: w354 -> [w375 w420]
              tunnel: w353 -> [w374 w418]
              tunnel: [_ w416] -> w352
              tunnel: [w370 _] -> w351
              tunnel: [_ w412] -> w350
              tunnel: w349 -> [w365 w405]
              tunnel: w348 -> [w358 _]
              tunnel: w347 -> [w362 _]
              frame #0 {
                n156 = for {
                  tunnel: w369 -> [w399] mode=indexing
                  tunnel: w375 -> [w392]
                  tunnel: w374 -> [w402]
                  tunnel: [w397] -> w373 mode=indexing
                  tunnel: [w393] -> w370 mode=indexing
                  tunnel: [w395] -> w364 mode=indexing
                  i -> [w401]
                  n157 = Increment(x=w401) -> (x+1=w400:i32)
                  n158 = local read "Polynomial Coefficients"() -> (w403:dbl[])
                  n159 = call "Polynomial_convert.vi"("Calib constants"=w403, "Voltage"=w400) -> ("Eng Values"=w393:dbl)  [unwired: 4 in]
                  n160 = Subtract(x=w399, y=w393) -> (x-y=w391:dbl[])
                  n161 = call "Puff_Stats_Low.vi"("Puff release time (s)"=w402, "Concentrations"=w391, "Time (s)"=w392) -> ("Stats"=w394:dbl[])  [unwired: 8 in]
                  n162 = Index Array(array=w394, index #1=1 ("index"), index #2=2 ("index")) -> (element #1=w397:dbl, element #2=w395:dbl)
                }
                n163 = for {
                  tunnel: w373 -> [w381] mode=indexing
                  tunnel: [w381] -> w368 mode=indexing if=w382
                  n164 = Less Than 0?(x=w381) -> (x < 0?=w382:bool)
                }
                n165 = Negate(x=w368) -> (-x=w367:dbl[])
                n166 = Build Array (concatenate)(w368, w367) -> (w366:dbl[])
                n167 = Empty Array?(array=w366) -> (empty?=w371:bool)
                n168 = case shown="False" w371 {
                  tunnel: [w377 0.0] -> w372
                  tunnel: w366 -> [w379 _]
                  tunnel: w365 -> [w376 _]
                  frame False {
                    n169 = call <vilib>:"Std Deviation and Variance.vi"("X"=w379) -> ("standard deviation"=w378:dbl)  [unwired: 1 in, 2 out]
                    n170 = Multiply(x=w378, y=w376) -> (x*y=w377:dbl)
                  }
                  frame True {
                  }
                }
                "Initial Minimum Dose" <- w372
                n171 = for {
                  tunnel: w364 -> [w384] mode=indexing
                  tunnel: w373 -> [w390] mode=indexing
                  tunnel: w372 -> [w389]
                  tunnel: [w384] -> w363 mode=indexing if=w387
                  tunnel: w358 -> [w386]
                  tunnel: w362 -> [w383]
                  n172 = In Range and Coerce(upper limit=w386, x=w384, lower limit=w383) -> (In Range?=w385:bool)  [unwired: 1 out]
                  n173 = Greater?(x=w390, y=w389) -> (0:w388:bool)
                  n174 = Compound Arithmetic op=AND(w388, w385) -> (w387:bool)
                }
                n175 = call-poly <vilib>:"Mean.vi"("X"=w363) -> ("mean"=w360:dbl)  [unwired: 1 out]
                n176 = Multiply(x=w358, y=0.6) -> (x*y=w357:dbl)
                n177 = Not A Number/Path/Refnum?(number/path/refnum=w360) -> (NaN/Path/Refnum?=w361:bool)
                n178 = Select(t=w357, s=w361, f=w360) -> (s? t:f=w359:dbl)
                "Initial Time of Flight" <- w359
                "Max Flight Time (s)" <- w358
              }
              frame #1 {
                n179 = for {
                  tunnel: w415 -> [w440] mode=indexing
                  tunnel: w420 -> [w439]
                  tunnel: w418 -> [w437]
                  tunnel: w419 -> [w436] mode=indexing
                  tunnel: w417 -> [w438]
                  tunnel: [w435] -> w416 mode=indexing
                  tunnel: [w432] -> w406 mode=indexing
                  shift-right: [w431] -> w414
                  shift-left: _ -> [w429]
                  tunnel: [w428] -> w413
                  i -> [w428]
                  n180 = Subtract(x=w440, y=w436) -> (x-y=w430:dbl[])
                  n181 = case shown="Default" w428 {
                    tunnel: [w441 w442] -> w431
                    tunnel: w430 -> [w441 w444]
                    tunnel: w429 -> [_ w443]
                    frame 0 {
                    }
                    frame Default {
                      n182 = Add(x=w444, y=w443) -> (x+y=w442:dbl[])
                    }
                  }
                  n183 = call "Puff_Stats.vi"("Puff release time (s)"=w437, "Initial Time of Flight"=w438, "Concentrations"=w430, "Time (s)"=w439) -> ("Stats Values"=w434:dbl[])  [unwired: 3 in, 4 out]
                  n184 = Build Array (concatenate)(w434, w436) -> (w435:dbl[])
                  n185 = Index Array(array=w434, index=1) -> (element=w432:dbl)
                }
                n186 = Increment(x=w413) -> (x+1=w411:i32)
                n187 = for {
                  tunnel: w406 -> [w426] mode=indexing
                  tunnel: [w426] -> w409 mode=indexing if=w427
                  n188 = Less Than 0?(x=w426) -> (x < 0?=w427:bool)
                }
                n189 = Divide(x=w414, y=w411) -> (x/y=w412:dbl[])
                n190 = Negate(x=w409) -> (-x=w408:dbl[])
                n191 = Build Array (concatenate)(w409, w408) -> (w407:dbl[])
                n192 = Empty Array?(array=w407) -> (empty?=w410:bool)
                n193 = case shown="False" w410 {
                  tunnel: [w422 0.0] -> w404
                  tunnel: w407 -> [w424 _]
                  tunnel: w405 -> [w421 _]
                  frame False {
                    n194 = call <vilib>:"Std Deviation and Variance.vi"("X"=w424) -> ("standard deviation"=w423:dbl)  [unwired: 1 in, 2 out]
                    n195 = Multiply(x=w423, y=w421) -> (x*y=w422:dbl)
                  }
                  frame True {
                  }
                }
                "Minimum Dose" <- w404
              }
            }
          }
        }
      }
      frame #6 {
        n196 = local read "Minimum Dose"() -> (w457:dbl)
        n197 = case shown="True" w465 {
          tunnel: w458 -> [_ w490]
          tunnel: w466 -> [_ w489]
          tunnel: w464 -> [_ w488]
          tunnel: [dbl[] [] w487] -> w463
          tunnel: w462 -> [w468 w486]
          tunnel: [w468 w485] -> w461
          tunnel: w460 -> [_ w484]
          tunnel: w459 -> [_ w483]
          tunnel: w457 -> [_ w482]
          tunnel: w456 -> [_ w481]
          tunnel: w455 -> [_ w480]
          tunnel: w453 -> [_ w479]
          tunnel: w454 -> [_ w478]
          tunnel: w452 -> [_ w477]
          tunnel: w451 -> [_ w476]
          tunnel: w450 -> [_ w475]
          tunnel: w449 -> [w467 w474]
          tunnel: [w467 w473] -> w448
          tunnel: w447 -> [_ w472]
          tunnel: w446 -> [_ w471]
          tunnel: w445 -> [_ w470]
          frame False {
          }
          frame True {
            # "Below"
            # "No"
            # "Value"
            # "Name"
            # "T"
            # "V"
            n198 = stacked-sequence {
              seq-local: [_ w528 _ _ _ _] -> [_ _ _ _ w670 _]
              seq-local: [_ w527 _ _ _ _] -> [_ _ _ _ w667 _]
              seq-local: [_ _ w563 _ _ _] -> [_ _ _ _ w638 _]
              seq-local: [_ _ w562 _ _ _] -> [_ _ _ _ w639 _]
              seq-local: [w504 _ _ _ _ _] -> [_ w526 _ _ w664 _]
              seq-local: [w503 _ _ _ _ _] -> [_ _ _ _ w637 _]
              seq-local: [w502 _ _ _ _ _] -> [_ _ _ _ w635 _]
              seq-local: [_ _ _ _ w662 _] -> [_ _ _ _ _ w683]
              seq-local: [_ _ _ _ w661 _] -> [_ _ _ _ _ w682]
              seq-local: [w501 _ _ _ _ _] -> [_ _ _ _ _ _]
              seq-local: [_ w521 _ _ _ _] -> [_ _ _ _ w649 _]
              seq-local: [w493 _ _ _ _ _] -> [_ _ _ _ w641 _]
              seq-local: [w491 _ _ _ _ _] -> [_ _ _ _ w646 _]
              seq-local: [_ _ w564 _ _ _] -> [_ _ _ w585 _ _]
              seq-local: [_ _ _ w609 _ _] -> [_ _ _ _ w636 _]
              seq-local: [_ _ _ w603 _ _] -> [_ _ _ _ w634 _]
              tunnel: w490 -> [w498 w531 _ _ _ _]
              tunnel: w489 -> [_ _ _ _ _ _]
              tunnel: w488 -> [_ _ w571 w588 _ _]
              tunnel: [_ w525 _ _ _ _] -> w487
              tunnel: w486 -> [_ _ _ _ _ w671]
              tunnel: [_ _ _ _ _ w681] -> w485
              tunnel: w484 -> [_ _ _ _ _ w684]
              tunnel: w483 -> [_ _ _ _ w660 _]
              tunnel: w482 -> [w500 _ _ _ w656 _]
              tunnel: w481 -> [_ _ w568 _ _ _]
              tunnel: w480 -> [w497 _ _ _ _ _]
              tunnel: w479 -> [w495 _ _ _ _ _]
              tunnel: w478 -> [_ _ _ _ w645 _]
              tunnel: w477 -> [_ _ _ _ _ _]
              tunnel: w476 -> [_ _ _ _ _ _]
              tunnel: w475 -> [_ _ _ w592 _ _]
              tunnel: w474 -> [_ _ _ w607 _ _]
              tunnel: [_ _ _ w606 _ _] -> w473
              tunnel: w472 -> [_ _ _ w593 _ _]
              tunnel: w471 -> [_ _ _ w608 _ _]
              tunnel: w470 -> [_ _ _ w594 _ _]
              frame #0 {
                n199 = Index Array(array=w498, index (col)=1 ("disabled index (col)")) -> (element=w505:dbl[])  [unwired: 1 in]
                n200 = Index Array(array=w498, index (col)=2 ("disabled index (col)")) -> (element=w496:dbl[])  [unwired: 1 in]
                n201 = for {
                  tunnel: w505 -> [w509] mode=indexing
                  tunnel: [w518] -> w503 mode=indexing
                  tunnel: [w517] -> w502 mode=indexing
                  tunnel: [w512] -> w504 mode=indexing
                  tunnel: [w509] -> w501 mode=indexing
                  tunnel: w500 -> [w516]
                  tunnel: w497 -> [w515]
                  tunnel: w496 -> [w513] mode=indexing
                  tunnel: w495 -> [w511]
                  tunnel: [w509] -> w494 mode=indexing if=w510
                  tunnel: [w507] -> w492 mode=indexing if=w508
                  i -> [w520]
                  n202 = Increment(x=w520) -> (x+1=w507:i32)
                  n203 = In Range and Coerce(upper limit=w515, x=w513, lower limit=w511) -> (In Range?=w514:bool)  [unwired: 1 out]
                  n204 = Greater?(x=w509, y=w516) -> (0:w508:bool)
                  n205 = Format Into String(format string="Puff %d:Dose (ppm s)", w507) -> (resulting string=w517:string)  [unwired: 2 in, 1 out]
                  n206 = call "Number_2_string.vi"("number"=w509) -> ("String"=w518:string)  [unwired: 1 in]
                  n207 = Not(x=w508) -> (.not. x?=w510:bool)
                  n208 = And(x=w508, y=w514) -> (x .and. y?=w512:bool)
                }
                n209 = Array Size(array=w492) -> (size(s)=w491:i32)
                n210 = call-poly <vilib>:"Mean.vi"("X"=w494) -> ("mean"=w493:dbl)  [unwired: 1 out]
                "Av Dose below Threshold" <- w493
              }
              frame #1 {
                w524 = bool[] [TRUE, TRUE, FALSE, FALSE, TRUE]  # Use All Puffs?
                w529 = string[] ["(s)", "(ppm s)", "(s)", "(s)", "(ppm)"]  # Units
                w530 = string[] ["Puff Length", "Dose", "T_flight", "Sigma_T_flight", "Puff_Bkgnd"]  # Quantity
                n211 = Array Size(array=w531) -> (size(s)=w533:i32[])
                n212 = Index Array(array=w533) -> (element #2=w532:i32)  [unwired: 2 in, 1 out]
                n213 = for {
                  N: w532 -> [_]
                  tunnel: w531 -> [w553]
                  tunnel: w530 -> [w545] mode=indexing
                  tunnel: w529 -> [w544] mode=indexing
                  tunnel: [w541] -> w528 mode=concatenating
                  tunnel: [w540] -> w527 mode=concatenating
                  tunnel: w526 -> [w538]
                  tunnel: [w537] -> w525 mode=indexing
                  tunnel: w524 -> [w536] mode=indexing
                  tunnel: [w534] -> w523 mode=indexing
                  i -> [w552]
                  n214 = Index Array(array=w553, index (col)=w552) -> (element=w539:dbl[])  [unwired: 1 in]
                  n215 = case shown="False" w536 {
                    tunnel: w539 -> [w556 w561]
                    tunnel: [w555 w561] -> w535
                    tunnel: w538 -> [w554 _]
                    frame False {
                      n216 = for {
                        tunnel: w556 -> [w560] mode=indexing
                        tunnel: [w560] -> w555 mode=indexing if=w557
                        tunnel: w554 -> [w558] mode=indexing
                        n217 = Not A Number/Path/Refnum?(number/path/refnum=w560) -> (NaN/Path/Refnum?=w559:bool)
                        n218 = Compound Arithmetic op=AND(w558, invert w559) -> (w557:bool)
                      }
                    }
                    frame True {
                    }
                  }
                  n219 = Concatenate Strings(w545, ":Mean " ("string"), w544) -> (w542:string)
                  n220 = Concatenate Strings(w545, ":St_Dev " ("string"), w544) -> (w543:string)
                  n221 = Array Size(array=w535) -> (size(s)=w534:i32)
                  n222 = call <vilib>:"Std Deviation and Variance.vi"("X"=w535, "Weighting (Sample)"=enum16{"Sample", "Population"}."Sample") -> ("mean"=w537:dbl, "standard deviation"=w550:dbl)  [unwired: 1 out]
                  n223 = call "Number_2_string.vi"("number"=w537) -> ("String"=w549:string)  [unwired: 1 in]
                  n224 = call "Number_2_string.vi"("number"=w550) -> ("String"=w548:string)  [unwired: 1 in]
                  n225 = Build Array(w542, w543) -> (w540:string[])
                  n226 = Build Array(w549, w548) -> (w541:string[])
                }
                n227 = Index Array(array=w523, index=2) -> (element=w521:i32)
              }
              frame #2 {
                w567 = FALSE  # Downsample Puff?
                n228 = case shown="True" w567 {
                  tunnel: w571 -> [w574 w579]
                  tunnel: [w574 w577] -> w570
                  tunnel: [w573 w576] -> w569
                  tunnel: w568 -> [w573 w575]
                  frame False {
                  }
                  frame True {
                    n229 = Array Size(array=w575) -> (size(s)=w580:i32)
                    n230 = Divide(x=w580, y=500) -> (x/y=w582:dbl)
                    n231 = Array Subset(array=w579, length=w580) -> (w578:dbl[])  [unwired: 1 in]
                    n232 = To Long Integer(number=w582) -> (32bit integer=w581:i32)
                    n233 = call "Downsampler.vi"("Input Array"=w575, "Averaging samples"=w581) -> ("Downsampled Array"=w576:dbl[])  [unwired: 1 out]
                    n234 = call "Downsampler.vi"("Input Array"=w578, "Averaging samples"=w581) -> ("Downsampled Array"=w577:dbl[])  [unwired: 1 out]
                  }
                }
                n235 = call "Puff_Analysis_AN.vi"("Input Own Peak Value?"=FALSE, "Concentration"=w569, "Time"=w570) -> ("End Index"=→"End Index":i32, "Start Index"=→"Start Index":i32, "Channel Values"=w562:string[], "Channel Names"=w563:string[], "Final Peak"=w564:dbl)  [unwired: 4 in]
              }
              frame #3 {
                n236 = Array Subset(array=w593, index (col)=w592) -> (w591:dbl[][])  [unwired: 3 in]
                n237 = Array Size(array=w591) -> (size(s)=w590:i32[])
                n238 = Index Array(array=w590, index=1) -> (element=w586:i32)
                n239 = Array Subset(array=w588, length=w586) -> (w587:dbl[])  [unwired: 1 in]
                n240 = for {
                  tunnel: w591 -> [w626] mode=indexing
                  tunnel: w587 -> [w624]
                  tunnel: w592 -> [_]
                  shift-right: [w628] -> w611
                  shift-left: _ -> [w629]
                  tunnel: [w627] -> w610
                  tunnel: [w621] -> w603
                  tunnel: w608 -> [_]
                  tunnel: w594 -> [w625] mode=indexing
                  tunnel: w585 -> [w620]
                  i -> [w627]
                  n241 = Subtract(x=w626, y=w625) -> (x-y=w623:dbl[])
                  n242 = call "Double Exponential Decay Fit.vi"("Peak Value"=w620, "Y"=w623, "X"=w624) -> ("Parameter Names"=w621:string[], "best fit parameters"=w622:dbl[])  [unwired: 6 in, 1 out]
                  n243 = case shown="Default" w627 {
                    tunnel: w622 -> [w630 w633]
                    tunnel: w629 -> [_ w632]
                    tunnel: [w630 w631] -> w628
                    frame 0 {
                    }
                    frame Default {
                      n244 = Add(x=w633, y=w632) -> (x+y=w631:dbl[])
                    }
                  }
                }
                n245 = Array Subset(array=w588, index=w592) -> (w596:dbl[])  [unwired: 1 in]
                n246 = Increment(x=w610) -> (x+1=w605:i32)
                n247 = Array Size(array=w603) -> (size(s)=w602:i32)
                n248 = Divide(x=w611, y=w605) -> (x/y=w600:dbl[])
                n249 = Index Array(array=w600) -> (element #1=w598:dbl, element #5=w584:dbl)  [unwired: 5 in, 3 out]
                n250 = Negate(x=w598) -> (-x=w599:dbl)
                n251 = for {
                  N: w586 -> [_]
                  tunnel: w588 -> [w619] mode=indexing
                  tunnel: w599 -> [w618]
                  tunnel: w585 -> [w616]
                  tunnel: w584 -> [w613]
                  tunnel: [w612] -> w597 mode=indexing
                  n252 = Divide(x=w619, y=w618) -> (x/y=w617:dbl)
                  n253 = Exponential(1:w617) -> (0:w615:dbl)
                  n254 = Multiply(x=w615, y=w616) -> (x*y=w614:dbl)
                  n255 = Add(x=w614, y=w613) -> (x+y=w612:dbl)
                }
                n256 = Array Subset(array=w600, length=w602) -> (w601:dbl[])  [unwired: 1 in]
                n257 = Number To Fractional String(number=w601, precision (6)=i16 3) -> (F-format string=w609:string[])  [unwired: 2 in]
                n258 = Bundle(w596, w597) -> (w595:cluster{dbl[], dbl[]})  [unwired: 1 in]
                n259 = Build Array (concatenate)(w607, w595) -> (w606:cluster{dbl[], dbl[]}[])
              }
              frame #4 {
                n260 = Array Size(array=w664) -> (size(s)=w665:i32)
                n261 = Array Max & Min(array=w660) -> (max value=w659:dbl)  [unwired: 3 out]
                n262 = Number To Fractional String(number=w659, precision (6)=i16 2) -> (F-format string=w652:string)  [unwired: 2 in]
                n263 = Number To Fractional String(number=w656, precision (6)=i16 4) -> (F-format string=w653:string)  [unwired: 2 in]
                n264 = Number To Fractional String(number=w641, precision (6)=i16 4) -> (F-format string=w640:string)  [unwired: 2 in]
                n265 = Number To Decimal String(number=w646) -> (decimal integer string=w663:string)  [unwired: 1 in]
                n266 = Number To Decimal String(number=w649) -> (decimal integer string=w650:string)  [unwired: 1 in]
                n267 = Number To Fractional String(number=w645, precision (6)=i16 1) -> (F-format string=w643:string)  [unwired: 2 in]
                n268 = Number To Decimal String(number=w665) -> (decimal integer string=w669:string)  [unwired: 1 in]
                n269 = Build Array (concatenate)(w667, "Number Of Puffs:Analysed" ("format string"), "Number Of:Non Zero Puffs" ("format string"), "Number Of Puffs:to get T_flight" ("format string"), "Threshold:St Dev" ("format string"), "Minium Dose:Threshold" ("format string"), "Av Dose:Below Threshold" ("format string"), "Max:Voltage" ("format string"), w638, w634, w635) -> (w662:string[])
                n270 = Build Array (concatenate)(w670, w669, w663, w650, w643, w653, w640, w652, w639, w636, w637) -> (w661:string[])
              }
              frame #5 {
                w678 = ":" ("string")
                n271 = Unbundle By Name(w671) -> ("Inst name"=w677:string)
                n272 = case shown="False" w684 {
                  tunnel: w683 -> [w691 w697]
                  tunnel: w682 -> [w690 w694]
                  tunnel: [w691 w693] -> w680
                  tunnel: [w690 w692] -> w673
                  frame False {
                  }
                  frame True {
                    n273 = local read "Output:Data File:Location"() -> (w695:string)
                    n274 = Build Array (concatenate)(w697, "Output Data File:Location") -> (w693:string[])
                    n275 = Build Array (concatenate)(w694, w695) -> (w692:string[])
                  }
                }
                n276 = Match Pattern(string=w677, regular expression=w678) -> (before substring=w676:string)  [unwired: 1 in, 3 out]
                n277 = Concatenate Strings(w676, w678) -> (w679:string)
                n278 = for {
                  tunnel: w680 -> [w689] mode=indexing
                  tunnel: w679 -> [w688]
                  tunnel: [w687] -> w674 mode=indexing
                  tunnel: w673 -> [w686] mode=indexing
                  tunnel: [w685] -> w675 mode=indexing
                  n279 = Concatenate Strings(w688, w689) -> (w687:string)
                  n280 = Build Array(w687, w686) -> (w685:string[])
                }
                "Table Control" <- w675
                n281 = Build Array(w674, w673) -> (w672:string[][])
                n282 = call "Update Metadata channels.vi"("Metadata Values"=w673, "Metadata Names"=w674, "Analysis info Cluster in"=w671) -> ("Analysis info Cluster out"=w681:T2)
                n283 = Transpose 2D Array(2D array=w672) -> ()  [unwired: 1 out]
              }
            }
          }
        }
        "Analysis info Cluster out" <- w461
        "XY Graph" <- w448
      }
      frame #7 {
        n284 = Index Array(array=w708, index (col)=1 ("disabled index (col)")) -> (element=w706:dbl[])  [unwired: 1 in]
        n285 = Index Array(array=w698, index (col)=1 ("disabled index (col)")) -> (element=w701:dbl[])  [unwired: 1 in]
        n286 = Array Size(array=w706) -> (size(s)=w707:i32)
        n287 = for {
          N: w707 -> [_]
          tunnel: [w709] -> w700 mode=indexing
          i -> [w711]
          n288 = Add(x=1.0, y=w711) -> (x+y=w709:dbl)
        }
        n289 = Bundle(w700, w706) -> (w703:cluster{dbl[], dbl[]})  [unwired: 1 in]
        n290 = Bundle(w700, w701) -> (w699:cluster{dbl[], dbl[]})  [unwired: 1 in]
        n291 = Build Array(w699, w703) -> (→"Dose per Puff":cluster{dbl[], dbl[]}[])
      }
      frame #8 {
        n292 = case shown="True" w727 {
          tunnel: w729 -> [_ w747]
          tunnel: w718 -> [_ w746]
          tunnel: w728 -> [_ w745]
          tunnel: w726 -> [_ w744]
          tunnel: w725 -> [_ w743]
          tunnel: w724 -> [_ w742]
          tunnel: w723 -> [_ w741]
          tunnel: w722 -> [_ w740]
          tunnel: w721 -> [_ w739]
          tunnel: [w730 w737] -> w720
          tunnel: w715 -> [w730 w738]
          tunnel: w719 -> [_ w736]
          tunnel: w717 -> [_ w735]
          tunnel: w716 -> [_ w734]
          tunnel: w714 -> [_ w733]
          tunnel: w713 -> [_ w732]
          tunnel: w712 -> [_ w731]
          frame False {
          }
          frame True {
            # "Len"
            # "Start"
            n293 = stacked-sequence {
              seq-local: [_ _ _ w859 _] -> [_ _ _ _ w933]
              seq-local: [_ w753 _ _ _] -> [_ _ _ w856 _]
              seq-local: [_ _ _ w855 _] -> [_ _ _ _ w931]
              seq-local: [_ _ w844 _ _] -> [_ _ _ w852 w929]
              seq-local: [_ _ w843 _ _] -> [_ _ _ w851 w928]
              seq-local: [_ _ w842 _ _] -> [_ _ _ w853 w927]
              seq-local: [w748 _ _ _ _] -> [_ w756 _ _ w926]
              seq-local: [_ _ w839 _ _] -> [_ _ _ w849 _]
              tunnel: w747 -> [w749 _ _ _ _]
              tunnel: w746 -> [_ w758 _ _ _]
              tunnel: w745 -> [_ w759 _ w862 w935]
              tunnel: w741 -> [_ _ _ w860 w936]
              tunnel: w744 -> [_ _ _ w861 w934]
              tunnel: w743 -> [_ _ _ w858 _]
              tunnel: w742 -> [_ w757 _ _ _]
              tunnel: w740 -> [_ w755 _ _ _]
              tunnel: w739 -> [_ _ _ w857 w932]
              tunnel: w738 -> [_ w754 _ _ _]
              tunnel: [_ _ _ _ w930] -> w737
              tunnel: w736 -> [_ _ w847 w854 _]
              tunnel: w735 -> [w750 _ _ w850 _]
              tunnel: w734 -> [_ _ _ _ w925]
              tunnel: w733 -> [_ w752 _ _ _]
              tunnel: w732 -> [_ _ _ _ _]
              tunnel: w731 -> [_ w751 _ w848 w924]
              frame #0 {
                n294 = Build Array (concatenate)(w750, w749) -> (w748:dbl[][])
              }
              frame #1 {
                n295 = case shown="False" w752 {
                  tunnel: w759 -> [_ w786]
                  tunnel: w758 -> [_ w785]
                  tunnel: w757 -> [_ w773]
                  tunnel: w756 -> [_ w772]
                  tunnel: w755 -> [_ w764]
                  tunnel: w754 -> [w760 w763]
                  tunnel: [w760 w762] -> w753
                  tunnel: w751 -> [_ w761]
                  frame False {
                  }
                  frame True {
                    w766 = string[] [] ("Extra Ch Names")
                    w770 = "\r\n"
                    w776 = ""
                    n296 = Bundle By Name(cluster=w761, "Initial Header String"="", "File Path"=w764, "Extra Ch Names"=w766, "Extra Ch Values"=w766) -> (w765:T1)
                    n297 = Array Size(array=w772) -> (size(s)=w798:i32[])
                    n298 = Index Array(array=w798) -> (element #1=w777:i32, element #2=w778:i32)  [unwired: 2 in]
                    n299 = for {
                      N: w778 -> [_]
                      tunnel: w772 -> [w813]
                      tunnel: w777 -> [w811]
                      tunnel: [w810] -> w779 mode=indexing
                      i -> [w812]
                      n300 = for {
                        N: w811 -> [_]
                        tunnel: w813 -> [w822]
                        tunnel: w812 -> [w821]
                        tunnel: [w814] -> w810 mode=indexing
                        i -> [w820]
                        n301 = Index Array(array=w822, index (row)=w820, index (col)=w821) -> (element=w815:dbl)
                        n302 = Equal To 0?(x=w820) -> (x = 0?=w819:bool)
                        n303 = Select(t=i16 3, s=w819, f=i16 1 ("precision (6)")) -> (s? t:f=w816:i16)
                        n304 = Number To Fractional String(number=w815, precision (6)=w816) -> (F-format string=w814:string)  [unwired: 2 in]
                      }
                    }
                    n305 = Build Array (concatenate)(w763, w765) -> (w762:T1[])
                    n306 = for {
                      N: w778 -> [_]
                      tunnel: w786 -> [w827] mode=indexing
                      tunnel: [w826] -> w789 mode=indexing
                      n307 = call "Number_2_string.vi"("number"=w827) -> ("String"=w826:string)  [unwired: 1 in]
                    }
                    n308 = for {
                      N: w777 -> [_]
                      tunnel: [w830] -> w783 mode=indexing
                      tunnel: [""] -> w787 mode=indexing
                      i -> [w828]
                      n309 = Format Into String(format string="Puff_%d", w828) -> (resulting string=w830:string)  [unwired: 2 in, 1 out]
                    }
                    n310 = Build Array (concatenate)(w776, "Puff_Length (s)", "Puff_Dose (ppm s)", "T_flight (s)", "Sigma_T_flight (s)", "Bkgnd_Value", w776, "Time (s)", w789) -> (w797:string[])
                    n311 = Replace Array Subset(array=w783, new element="Averaged Puff", index=0) -> (w782:string[])
                    n312 = Build Array (concatenate)(w773, w785) -> (w784:dbl[][])
                    n313 = Transpose 2D Array(2D array=w784) -> (transposed array=w800:dbl[][])
                    n314 = for {
                      tunnel: w800 -> [w833] mode=indexing
                      tunnel: [w832] -> w799 mode=indexing
                      n315 = for {
                        tunnel: w833 -> [w835] mode=indexing
                        tunnel: [w834] -> w832 mode=indexing
                        n316 = call "Number_2_string.vi"("number"=w835) -> ("String"=w834:string)  [unwired: 1 in]
                      }
                    }
                    n317 = case shown="True" "Puff Stats only?" {
                      tunnel: w799 -> [w804 w809]
                      tunnel: [w803 w808] -> w796
                      tunnel: w787 -> [w802 w807]
                      tunnel: w782 -> [w801 w806]
                      tunnel: w779 -> [_ w805]
                      frame True {
                        n318 = Build Array (concatenate)(w801, w804, w802) -> (w803:string[][])
                      }
                      frame False {
                        n319 = Build Array (concatenate)(w806, w809, w807, w806, w805) -> (w808:string[][])
                      }
                    }
                    n320 = for {
                      tunnel: w797 -> [w823] mode=indexing
                      tunnel: w796 -> [w825] mode=indexing
                      tunnel: [w824] -> w795 mode=indexing
                      n321 = Build Array (concatenate)(w823, w825) -> (w824:string[])
                    }
                    n322 = Array To Spreadsheet String(array=w795, 3:"%s" ("format string")) -> (spreadsheet string=w768:string)  [unwired: 1 in]
                    n323 = Concatenate Strings(w770, w770, w768) -> (w769:string)
                    n324 = call "Write_File_Simple.vi"("append to file? (new file:F)"=FALSE, "character string"=w769, "file path"=w764) -> ()  [unwired: 2 out]
                  }
                }
              }
              frame #2 {
                n325 = global read "Dynamic_call_global.ph.vi" "Initial Plug Ins Extra"() -> (w838:string[])
                n326 = global read "Dynamic_call_global.ph.vi" "Initial Plug Ins"() -> (w837:string[])
                n327 = Build Array (concatenate)(w837, w838) -> (w836:string[])
                n328 = Search 1D Array(1D array=w836, element="Move_Trav_while_Meas_Blocks.vi") -> (index of element=w840:i32)  [unwired: 1 in]
                n329 = Greater Or Equal To 0?(x=w840) -> (x >= 0?=w839:bool)
                n330 = local read "Start Index"() -> (w844:i32)
                n331 = local read "End Index"() -> (w845:i32)
                n332 = Subtract(x=w845, y=w844) -> (x-y=w843:i32)
                n333 = Divide(x=w843, y=w847) -> (x/y=w846:dbl)
                n334 = To Long Integer(number=w846) -> (32bit integer=w842:i32)
              }
              frame #3 {
                n335 = case shown="True" w858 {
                  tunnel: w862 -> [_ w887]
                  tunnel: w861 -> [_ w902]
                  tunnel: w860 -> [_ w901]
                  tunnel: [w864 w890] -> w859
                  tunnel: w857 -> [_ w888]
                  tunnel: w848 -> [_ w867]
                  tunnel: w856 -> [w863 w880]
                  tunnel: [w863 w879] -> w855
                  tunnel: w854 -> [_ _]
                  tunnel: w853 -> [_ w877]
                  tunnel: w852 -> [_ w876]
                  tunnel: w851 -> [_ w875]
                  tunnel: w850 -> [_ w872]
                  tunnel: w849 -> [_ w870]
                  frame False {
                    n336 = global read "Meas_global.vi" "Results file"() -> (w866:path)
                    n337 = Strip Path(path=w866) -> (name=w865:string)  [unwired: 1 out]
                    n338 = call "Add_filename_suffix.vi"("Filename"=w865) -> ("Base name"=w864:string)  [unwired: 1 in, 3 out]
                  }
                  frame True {
                    w884 = "\r\n"
                    w885 = string[] [] ("Extra Ch Names")
                    w909 = "\r\n"
                    n339 = global read "Meas_global.vi" "Results file"() -> (w907:path)
                    n340 = Strip Path(path=w907) -> (name=w896:string)  [unwired: 1 out]
                    n341 = global read "Meas_global.vi" "Raw data file"() -> (w906:path)
                    n342 = Array Subset(array=w887, index=w876, length=w875) -> (w905:dbl[])
                    n343 = Array Subset(array=w872, index=w876, length=w875) -> (w886:dbl[])
                    n344 = call "Add_filename_suffix.vi"("Filename"=w896) -> ("Base name"=w890:string)  [unwired: 1 in, 3 out]
                    n345 = call "Downsampler.vi"("Input Array"=w886, "Averaging samples"=w877) -> ("Downsampled Array"=w895:dbl[])  [unwired: 1 out]
                    n346 = call "Downsampler.vi"("Input Array"=w905, "Averaging samples"=w877) -> ("Downsampled Array"=w871:dbl[])  [unwired: 1 out]
                    n347 = Build Path(base path=w888, name or relative path="Average_Puff_files") -> (appended path=w897:path)
                    n348 = Strip Path(path=w906) -> (name=w899:string)  [unwired: 1 out]
                    n349 = call "Add_filename_suffix.vi"("Filename"=w899) -> ("Base name"=w903:string)  [unwired: 1 in, 3 out]
                    n350 = case shown="False" w870 {
                      tunnel: w871 -> [w919 w923]
                      tunnel: [w919 w921] -> w869
                      tunnel: [i16 3 ("precision (6)") i16 5 ("precision (6)")] -> w868
                      frame False {
                      }
                      frame True {
                        n351 = Index Array(array=w923) -> (element=w922:dbl)  [unwired: 1 in]
                        n352 = Subtract(x=w923, y=w922) -> (x-y=w921:dbl[])
                      }
                    }
                    n353 = Build Path(base path=w897, name or relative path=w890) -> (appended path=w898:path)
                    n354 = Format Into String(format string="_%s%s", initial string=w903, w902, w901) -> (resulting string=w900:string)  [unwired: 1 in, 1 out]
                    n355 = Concatenate Strings("Time (s)", "\t", "Av_Puff (ppm)") -> (w893:string)
                    n356 = Initialize Array("", 10) -> (w915:string[])
                    n357 = Build Path(base path=w898, name or relative path=w900) -> (appended path=w878:path)
                    n358 = Build Array(w869, w895) -> (w913:dbl[][])
                    n359 = call "Asterisk_header.vi"("Channel names"=w915) -> ("Header string"=w914:string)
                    n360 = Transpose 2D Array(2D array=w913) -> (transposed array=w911:dbl[][])
                    n361 = Number To Fractional String(number=w911, precision (6)=w868) -> (F-format string=w910:string[][])  [unwired: 2 in]
                    n362 = Concatenate Strings(w884, "*****This is a many rows per single point file*****", w884) -> (w882:string)
                    n363 = call "Create_directory_path.vi"("Path name"=w878) -> ("Path name Out"=w874:path)  [unwired: 2 in, 1 out]
                    n364 = Array To Spreadsheet String(array=w910, 3:"%s" ("format string")) -> (spreadsheet string=w908:string)  [unwired: 1 in]
                    n365 = Bundle By Name(cluster=w867, "Initial Header String"=w882, "File Path"=w874, "Extra Ch Names"=w885, "Extra Ch Values"=w885) -> (w881:T1)
                    n366 = Build Array (concatenate)(w881, w880) -> (w879:T1[])
                    n367 = Concatenate Strings(w909, w914, w893, w909, w909, w909, w908) -> (w873:string)
                    n368 = Write to Text File(file (use dialog)=w874, text=w873) -> ()  [unwired: 2 in, 3 out]
                  }
                }
              }
              frame #4 {
                n369 = case shown="True" w925 {
                  tunnel: w936 -> [_ w950]
                  tunnel: w935 -> [_ w949]
                  tunnel: w926 -> [_ w948]
                  tunnel: w934 -> [_ w947]
                  tunnel: w933 -> [_ w946]
                  tunnel: w932 -> [_ w945]
                  tunnel: w924 -> [_ w944]
                  tunnel: w931 -> [w937 w943]
                  tunnel: [w937 w941] -> w930
                  tunnel: w929 -> [_ w940]
                  tunnel: w928 -> [_ w939]
                  tunnel: w927 -> [_ w938]
                  frame False {
                  }
                  frame True {
                    n370 = for {
                      tunnel: w950 -> [w980]
                      tunnel: w949 -> [w982]
                      tunnel: w948 -> [w958] mode=indexing
                      tunnel: w947 -> [w973]
                      tunnel: w946 -> [w969]
                      tunnel: w945 -> [w968]
                      tunnel: w944 -> [w961]
                      tunnel: [w960] -> w942 mode=indexing
                      tunnel: w940 -> [w956]
                      tunnel: w939 -> [w955]
                      tunnel: w938 -> [w954]
                      i -> [w974]
                      w966 = "\r\n"
                      w985 = "\r\n"
                      n371 = Number To Decimal String(number=w974) -> (decimal integer string=w972:string)  [unwired: 1 in]
                      n372 = global read "Meas_global.vi" "Raw data file"() -> (w983:path)
                      n373 = Array Subset(array=w958, index=w956, length=w955) -> (w957:dbl[])
                      n374 = Array Subset(array=w982, index=w956, length=w955) -> (w981:dbl[])
                      n375 = Build Path(base path=w968, name or relative path="Individual_Puff_Files") -> (appended path=w971:path)
                      n376 = Strip Path(path=w983) -> (name=w976:string)  [unwired: 1 out]
                      n377 = call "Add_filename_suffix.vi"("Filename"=w976) -> ("Base name"=w979:string)  [unwired: 1 in, 3 out]
                      n378 = call "Downsampler.vi"("Input Array"=w957, "Averaging samples"=w954) -> ("Downsampled Array"=w991:dbl[])  [unwired: 1 out]
                      n379 = call "Downsampler.vi"("Input Array"=w981, "Averaging samples"=w954) -> ("Downsampled Array"=w992:dbl[])  [unwired: 1 out]
                      n380 = Initialize Array("", 10) -> (w998:string[])
                      n381 = Build Path(base path=w971, name or relative path=w969) -> (appended path=w977:path)
                      n382 = case shown="0" w974 {
                        tunnel: w980 -> [w1005 w1013]
                        tunnel: w974 -> [_ w1012]
                        tunnel: w979 -> [w1004 w1011]
                        tunnel: [w1003 w1010] -> w978
                        tunnel: w973 -> [w1002 w1008]
                        tunnel: ["Average" w1007] -> w962
                        tunnel: w972 -> [_ w1007]
                        frame 0 {
                          n383 = Format Into String(format string="_%s_Av%s", initial string=w1004, w1002, w1005) -> (resulting string=w1003:string)  [unwired: 1 in, 1 out]
                        }
                        frame 1, Default {
                          n384 = Format Into String(format string="_%s_%d%s", initial string=w1011, w1008, w1012, w1013) -> (resulting string=w1010:string)  [unwired: 1 in, 1 out]
                        }
                      }
                      n385 = call "Asterisk_header.vi"("Channel names"=w998) -> ("Header string"=w997:string)
                      n386 = Build Array(w992, w991) -> (w990:dbl[][])
                      n387 = Build Path(base path=w977, name or relative path=w976) -> (appended path=w975:path)
                      n388 = Concatenate Strings("Time (s)", "\t", "C (ppm)") -> (w993:string)
                      n389 = Transpose 2D Array(2D array=w990) -> (transposed array=w988:dbl[][])
                      n390 = Number To Fractional String(number=w988, precision (6)=i16 3) -> (F-format string=w986:string[][])  [unwired: 2 in]
                      n391 = Build Path(base path=w975, name or relative path=w978) -> (appended path=w953:path)
                      n392 = Build Array("Puff:Block:Number" ("element")) -> (w963:string[])
                      n393 = Concatenate Strings(w966, "*****This is a many rows per single point file*****", w966) -> (w965:string)
                      n394 = Build Array(w962) -> (w959:string[])
                      n395 = Array To Spreadsheet String(array=w986, 3:"%s" ("format string")) -> (spreadsheet string=w984:string)  [unwired: 1 in]
                      n396 = Concatenate Strings(w985, w997, w993, w985, w985, w985, w984) -> (w951:string)
                      n397 = call "Create_directory_path.vi"("Path name"=w953) -> ("Path name Out"=w952:path)  [unwired: 2 in, 1 out]
                      n398 = Bundle By Name(cluster=w961, "Initial Header String"=w965, "File Path"=w952, "Extra Ch Names"=w963, "Extra Ch Values"=w959) -> (w960:T1)
                      n399 = Write to Text File(file (use dialog)=w952, text=w951) -> ()  [unwired: 2 in, 3 out]
                    }
                    n400 = Build Array (concatenate)(w942, w943) -> (w941:T1[])
                  }
                }
              }
            }
          }
        }
      }
      frame #9 {
        n401 = Build Array("Row Number") -> (w1016:i32[])
        n402 = for {
          tunnel: w1016 -> [w1020]
          tunnel: w1015 -> [w1019] mode=indexing
          tunnel: [w1018] -> w1014 mode=indexing
          n403 = Bundle By Name(cluster=w1019, "Rows to Add"=w1020) -> (w1018:T1)
        }
        "File to Update" <- w1014
      }
    }
  }
